vi "getElement.vi"(7 "Type and Defaults":variant, 8 "error in":errorcluster, 9 "pathList":string[](array[string]), 10 "basePath in":string, 11 "JSON String":string="{\n  \"VersionHistory\": {\n    \"InitialAuthor\": \"ABC\",\n    \"DateCreated\": \"03:45:56 AM 22/02/2017\",\n    \"DatesModified\": [\n      \"03:45:56 AM 22/02/2017\",\n      \"03:45:56 AM 22/02/2017\",\n      \"03:45:56 AM 22/02/2017\"\n    ],\n    \"ModifiedBy\": [\n      \"DEF\",\n      \"GHI\",\n      \"JKL\"\n    ],\n    \"DocumentVersion\": \"2.1.2\",\n    \"ZenParamsSpecVersion\": \"3.2.1\"\n  },\n  \"SystemParameters\": {\n    \"SystemName\": \"Tiger\",\n    \"SystemID\": 123,\n    \"CustomerName\": \"TT\",\n    \"Location\": \"Bangalore\",\n    \"InstallationDate\": \"10-02-2017\",\n    \"NextServiceDate\": \"16-07-2017\",\n    \"ServiceHistory\": [\n      \"16-07-2016\",\n      \"16-08-2016\"\n    ],\n    \"CompatibleZenGage\": \"1.1\",\n    \"TotalNumberOfCameras\": 3,\n    \"NumberOfRacks\": 1,\n    \"SoftwareFeature\": {\n      \"comment_SoftwareFeatures\": \"//Software feature contains controls to Enable/Disable POST, Cp Cpk Report, Analytics, Data Logging and control to set value for Maximum Digital Zoom//\",\n      \"POSTEnable\": true,\n      \"CpCpkReportEnable\": true,\n      \"AnalyticsEnable\": true,\n      \"DataLoggingEnable\": true,\n      \"MaxDigitalZoom\": 5\n    },\n    \"GuideHorizontalPositioningEnable\": true,\n    \"comment_Sensor\": \"//Sensor section contains Name, Unique Id, Controller IO number and Triggering Edge of each sensor//\",\n    \"Sensor\": [\n      {\n        \"Name\": \"pqr\",\n        \"Id\": 1,\n        \"ControllerIONumber\": 12,\n        \"Edge\": \"FALLING\"\n      },\n      {\n        \"Name\": \"stu\",\n        \"Id\": 2,\n        \"ControllerIONumber\": 12,\n        \"Edge\": \"FALLING\"\n      },\n      {\n        \"Name\": \"vwx\",\n        \"Id\": 3,\n        \"ControllerIONumber\": 12,\n        \"Edge\": \"FALLING\"\n      }\n    ],\n    \"comment_Light\": \"//Light section contains Name, Unique Id, Type (Can be Bright field, Dark field, Back light, Front light, Diffuse light, Co-Axial diffuse etc.), Controller IO number and Level (HIGH or LOW) of each Light//\",\n    \"Light\": [\n      {\n        \"Name\": \"Light1\",\n        \"Id\": 1,\n        \"Type\": \"Back\",\n        \"ControllerIONumber\": 23,\n        \"Level\": \"HIGH\"\n      },\n      {\n        \"Name\": \"Light2\",\n        \"Id\": 2,\n        \"Type\": \"Front\",\n        \"ControllerIONumber\": 23,\n        \"Level\": \"HIGH\"\n      },\n      {\n        \"Name\": \"Light3\",\n        \"Id\": 3,\n        \"Type\": \"Back\",\n        \"ControllerIONumber\": 23,\n        \"Level\": \"HIGH\"\n      }\n    ],\n    \"comment_Camera\": \"//Camera section contains Camera Id, Type (Top, Side or Front), Model, Area of Interest (AOI), Trigger Mode, Controller IO Number, Triggering Edge, Pulse Width, Exposure Time in micro seconds, Interface Type (Allowed values are USB3, GigE, USB2), Gain in dB, Calibration details (Date and file path) of each camera//\",\n    \"Camera\": [\n      {\n        \"Id\": 1,\n        \"Type\": \"Top\",\n        \"Model\": \"Basler Ace 5MP\",\n        \"AOI\": [\n          12,\n          34,\n          56,\n          78\n        ],\n        \"TriggerMode\": \"External\",\n        \"ControllerIONumber\": 34,\n        \"Edge\": \"FALLING\",\n        \"PulseWidth\": 233,\n        \"ExposureTimeUSec\": 12,\n        \"InterfaceType\": \"USB3\",\n        \"GainIndB\": 6,\n        \"CalibrationDate\": \"12-01-2017\",\n        \"CalibrationFilePath\": \"C:\\\\Users\\\\veenaj\\\\Desktop\"\n      },\n      {\n        \"Id\": 2,\n        \"Type\": \"Side\",\n        \"Model\": \"Basler Ace 5MP\",\n        \"AOI\": [\n          12,\n          34,\n          56,\n          78\n        ],\n        \"TriggerMode\": \"External\",\n        \"ControllerIONumber\": 34,\n        \"Edge\": \"FALLING\",\n        \"PulseWidth\": 233,\n        \"ExposureTimeUSec\": 12,\n        \"InterfaceType\": \"USB3\",\n        \"GainIndB\": 6,\n        \"CalibrationDate\": \"12/04/17\",\n        \"CalibrationFilePath\": \"C:\\\\Desktop\\\\Calibration\"\n      },\n      {\n        \"Id\": 3,\n        \"Type\": \"Front\",\n        \"Model\": \"Basler Ace 5MP\",\n        \"AOI\": [\n          12,\n          34,\n          56,\n          78\n        ],\n        \"TriggerMode\": \"External\",\n        \"ControllerIONumber\": 34,\n        \"Edge\": \"FALLING\",\n        \"PulseWidth\": 233,\n        \"ExposureTimeUSec\": 12,\n        \"InterfaceType\": \"USB3\",\n        \"GainIndB\": 6,\n        \"CalibrationDate\": \"12/04/17\",\n        \"CalibrationFilePath\": \"C:\\\\Desktop\\\\Calibration\"\n      }\n    ]\n  },\n  \"PartParameters\": {\n    \"comment_PartParameters\": \"//Parts Parameters section includes Number of Parts configured and Parts List. Part List contains Name, Parallel Trigger Threads, Number of measurements and Measurement details//\",\n    \"NumberOfPartsConfigured\": 2,\n    \"PartsList\": [\n      {\n        \"Name\": \"ECU1511\",\n        \"comment_ParallelTriggerThreads\": \"//ParallelTriggerThreads contain Thread Name, Thread Id and Imaging Views. Combination of Camera and Light(s) is defined in Imaging View along with Sensor to Light Delay (in micro seconds), Light to Camera Trigger Delay, Light Pulse Width and Reference Co-ordinate system. Each Imaging View is given a Name and unique ImageId. Camera and Light(s) are accessed by their unique Ids.//\",\n        \"ParallelTriggerThreads\": [\n          {\n            \"ThreadName\": \"TopRack\",\n            \"ThreadId\": 1,\n            \"ImagingViews\": [\n              {\n                \"ImageId\": 1,\n                \"ViewName\": \"TopProfileView\",\n                \"CameraId\": 3,\n                \"LightIds\": [\n                  1,\n                  4,\n                  5\n                ],\n                \"SensorToLightDelayinUSec\": 12,\n                \"LightToCameraTriggerDelay\": 24,\n                \"LightPulseWidth\": 123,\n                \"ReferenceCoordSystem\": {\n                  \"Method\": [\n                    \"A\",\n                    \"B\",\n                    \"C\",\n                    \"D\",\n                    \"R\",\n                    \"V\"\n                  ],\n                  \"comment_RefROI\": \"//Reference ROI is cluster of Left, Top, Right, Bottom and Rotation values//\",\n                  \"ROI1\": [\n                    1014,\n                    95,\n                    1290,\n                    520,\n                    0\n                  ],\n                  \"ROI2\": [\n                    740,\n                    70,\n                    1040,\n                    340,\n                    0\n                  ],\n                  \"ROI3\": [\n                    1060,\n                    88,\n                    723,\n                    85,\n                    0\n                  ],\n                  \"Name\": \"FirstReference\"\n                }\n              },\n              {\n                \"ImageId\": 2,\n                \"ViewName\": \"TopLightView\",\n                \"CameraId\": 2,\n                \"LightIds\": [\n                  2,\n                  3,\n                  5\n                ],\n                \"SensorToLightDelayinUSec\": 12,\n                \"LightToCameraTriggerDelay\": 24,\n                \"LightPulseWidth\": 123,\n                \"ReferenceCoordSystem\": {\n                  \"Method\": [\n                    \"A\",\n                    \"B\",\n                    \"C\",\n                    \"D\",\n                    \"R\",\n                    \"V\"\n                  ],\n                  \"comment_RefROI\": \"//Reference ROI is cluster of Left, Top, Right, Bottom and Rotation values//\",\n                  \"ROI1\": [\n                    1014,\n                    95,\n                    1290,\n                    520,\n                    0\n                  ],\n                  \"ROI2\": [\n                    740,\n                    70,\n                    1040,\n                    340,\n                    0\n                  ],\n                  \"ROI3\": [\n                    1060,\n                    88,\n                    723,\n                    85,\n                    0\n                  ],\n                  \"Name\": \"FirstReference\"\n                }\n              }\n            ]\n          },\n          {\n            \"ThreadName\": \"BottomRack\",\n            \"ThreadId\": 2,\n            \"ImagingViews\": [\n              {\n                \"ImageId\": 1,\n                \"ViewName\": \"TopProfileView\",\n                \"CameraId\": 3,\n                \"LightIds\": [\n                  1,\n                  4,\n                  5\n                ],\n                \"SensorToLightDelayinUSec\": 12,\n                \"LightToCameraTriggerDelay\": 24,\n                \"LightPulseWidth\": 123,\n                \"ReferenceCoordSystem\": {\n                  \"Method\": [\n                    \"A\",\n                    \"B\",\n                    \"C\",\n                    \"D\",\n                    \"R\",\n                    \"V\"\n                  ],\n                  \"comment_RefROI\": \"//Reference ROI is cluster of Left, Top, Right, Bottom and Rotation values//\",\n                  \"ROI1\": [\n                    1014,\n                    95,\n                    1290,\n                    520,\n                    0\n                  ],\n                  \"ROI2\": [\n                    740,\n                    70,\n                    1040,\n                    340,\n                    0\n                  ],\n                  \"ROI3\": [\n                    1060,\n                    88,\n                    723,\n                    85,\n                    0\n                  ],\n                  \"Name\": \"FirstReference\"\n                }\n              },\n              {\n                \"ImageId\": 2,\n                \"ViewName\": \"TopLightView\",\n                \"CameraId\": 2,\n                \"LightIds\": [\n                  2,\n                  3,\n                  5\n                ],\n                \"SensorToLightDelayinUSec\": 12,\n                \"LightToCameraTriggerDelay\": 24,\n                \"LightPulseWidth\": 123,\n                \"ReferenceCoordSystem\": {\n                  \"Method\": [\n                    \"A\",\n                    \"B\",\n                    \"C\",\n                    \"D\",\n                    \"R\",\n                    \"V\"\n                  ],\n                  \"comment_RefROI\": \"//Reference ROI is cluster of Left, Top, Right, Bottom and Rotation values//\",\n                  \"ROI1\": [\n                    1014,\n                    95,\n                    1290,\n                    520,\n                    0\n                  ],\n                  \"ROI2\": [\n                    740,\n                    70,\n                    1040,\n                    340,\n                    0\n                  ],\n                  \"ROI3\": [\n                    1060,\n                    88,\n                    723,\n                    85,\n                    0\n                  ],\n                  \"Name\": \"FirstReference\"\n                }\n              }\n            ]\n          },\n          {\n            \"ThreadName\": \"DentIdentification\",\n            \"ThreadId\": 3,\n            \"ImagingViews\": [\n              {\n                \"ImageId\": 1,\n                \"ViewName\": \"TopProfileView\",\n                \"CameraId\": 3,\n                \"LightIds\": [\n                  1,\n                  4,\n                  5\n                ],\n                \"SensorToLightDelayinUSec\": 12,\n                \"LightToCameraTriggerDelay\": 24,\n                \"LightPulseWidth\": 123,\n                \"ReferenceCoordSystem\": {\n                  \"Method\": [\n                    \"A\",\n                    \"B\",\n                    \"C\",\n                    \"D\",\n                    \"R\",\n                    \"V\"\n                  ],\n                  \"comment_RefROI\": \"//Reference ROI is cluster of Left, Top, Right, Bottom and Rotation values//\",\n                  \"ROI1\": [\n                    23,\n                    78,\n                    99,\n                    25,\n                    0\n                  ],\n                  \"ROI2\": [\n                    67,\n                    97,\n                    43,\n                    9,\n                    0\n                  ],\n                  \"ROI3\": [\n                    45,\n                    88,\n                    723,\n                    85,\n                    0\n                  ],\n                  \"Name\": \"FirstReference\"\n                }\n              }\n            ]\n          }\n        ],\n        \"Number of Measurements\": 3,\n        \"comment_Measurements\": \"//Measurements section contains Name, Type, Enable, Algorithm Sequence, Calibration Co-efficients, User Correction Linearity Coefficients, User Correction Bias Coefficients, LSL, USL, LCL, UCL, Control Limits Violation Threshold, Specification Limits Violation Threshold, Overlay Options, Datalog Enable, Display Icon path for each Measurement//\",\n        \"Measurements\": [\n          {\n            \"Name\": \"CollarWidth\",\n            \"comment_Type\": \"//Type can be Linear or Angle//\",\n            \"Type\": \"Linear\",\n            \"Enable\": true,\n            \"comment_AlgorithmSequence\": \"//Particular Measurement may require sequence of Algorithms. ThreadId and ThreadImageId are mentioned in each Algorithm which corresponds to particular combination of Camera and Light Ids. Result of each Algorithm is stored in a variable and final result is calculated using Math Expression defined.//\",\n            \"AlgorithmSequence\": [\n              {\n                \"AlgoName\": \"MaxClamp\",\n                \"ThreadId\": 1,\n                \"ThreadImageId\": 2,\n                \"Option1\": \"\",\n                \"Option2\": \"\",\n                \"Option3\": \"\",\n                \"LocalRef\": {\n                  \"LocalCoordinateSystemEnable\": true,\n                  \"Method\": [\n                    \"A\",\n                    \"B\",\n                    \"C\",\n                    \"D\",\n                    \"R\",\n                    \"V\"\n                  ],\n                  \"comment_LocalRefROI\": \"//Local Reference ROI is cluster of Left, Top, Right, Bottom and Rotation values//\",\n                  \"ROIs\": [\n                    [\n                      23,\n                      78,\n                      99,\n                      25,\n                      0\n                    ],\n                    [\n                      67,\n                      97,\n                      43,\n                      9,\n                      0\n                    ],\n                    [\n                      45,\n                      88,\n                      723,\n                      85,\n                      0\n                    ]\n                  ],\n                  \"Name\": \"CollarWidthLocalReference\"\n                },\n                \"LocalROIs\": [\n                  [\n                    23,\n                    78,\n                    99,\n                    25,\n                    0\n                  ],\n                  [\n                    67,\n                    97,\n                    43,\n                    9,\n                    0\n                  ],\n                  [\n                    45,\n                    88,\n                    723,\n                    85,\n                    0\n                  ]\n                ],\n                \"comment_Overlay\": \"//OverlayOptions contain Text, Co ordinates, Angle in Degrees, Text Size and Text Color for Overlay//\",\n                \"OverlayOptions\": {\n                  \"OverlayEnable\": true,\n                  \"OverlayText\": \"Collar Width\",\n                  \"OverlayCoords\": [\n                    5,\n                    8\n                  ],\n                  \"OverlayAngle\": 56,\n                  \"OverlayTextSize\": 6,\n                  \"OverlayTextColor\": \"Red\"\n                },\n                \"ResultVariable\": \"M1\"\n              },\n              {\n                \"AlgoName\": \"MoveXYTable\",\n                \"XYDelta\": [\n                  56,\n                  -33.8\n                ]\n              },\n              {\n                \"AlgoName\": \"MaxClamp\",\n                \"ThreadId\": 1,\n                \"ThreadImageId\": 2,\n                \"Option1\": \"\",\n                \"Option2\": \"\",\n                \"Option3\": \"\",\n                \"LocalRef\": {\n                  \"LocalCoordinateSystemEnable\": true,\n                  \"Method\": [\n                    \"A\",\n                    \"B\",\n                    \"C\",\n                    \"D\",\n                    \"R\",\n                    \"V\"\n                  ],\n                  \"ROIs\": [\n                    [\n                      23,\n                      78,\n                      99,\n                      25,\n                      0\n                    ],\n                    [\n                      67,\n                      97,\n                      43,\n                      9,\n                      0\n                    ],\n                    [\n                      45,\n                      88,\n                      723,\n                      85,\n                      0\n                    ]\n                  ],\n                  \"Name\": \"CollarWidthLocalReference\"\n                },\n                \"LocalROIs\": [\n                  [\n                    23,\n                    78,\n                    99,\n                    25,\n                    0\n                  ],\n                  [\n                    67,\n                    97,\n                    43,\n                    9,\n                    0\n                  ],\n                  [\n                    45,\n                    88,\n                    723,\n                    85,\n                    0\n                  ]\n                ],\n                \"comment_Overlay\": \"//OverlayOptions contain Text, Co ordinates, Angle in Degrees, Text Size and Text Color for Overlay//\",\n                \"OverlayOptions\": {\n                  \"OverlayEnable\": true,\n                  \"OverlayText\": \"Collar Width\",\n                  \"OverlayCoords\": [\n                    5,\n                    8\n                  ],\n                  \"OverlayAngle\": 56,\n                  \"OverlayTextSize\": 6,\n                  \"OverlayTextColor\": \"Red\"\n                },\n                \"ResultVariable\": \"M2\"\n              },\n              {\n                \"Algorithm\": \"Math\",\n                \"MathExpression\": \"M2-M1\",\n                \"ResultVariable\": \"M3\"\n              }\n            ],\n            \"CalibrationCoefficients\": [\n              13,\n              8.7,\n              67.9\n            ],\n            \"UserCorrectionLinearityCoeff\": 45,\n            \"UserCorrectionBiasCoeff\": 56,\n            \"comment_LSL\": \"//Lower Specification Limit//\",\n            \"LSL\": 13.5,\n            \"comment_USL\": \"//Upper Specification Limit//\",\n            \"USL\": 15,\n            \"comment_LCL\": \"//Lower Control Limit//\",\n            \"LCL\": 13.5,\n            \"comment_UCL\": \"//Upper Control Limit//\",\n            \"UCL\": 15,\n            \"comment_ControlLimitsViolationThreshold\": \"//If 3 measurement results out of 1000, are crossing LCL and UCL then fail is detected//\",\n            \"ControlLimitsViolationThreshold\": [\n              3,\n              1000\n            ],\n            \"comment_SpecificationLimitsViolationThreshold\": \"//If 5 measurement results out of 5000, are crossing LSL and USL then fail is detected//\",\n            \"SpecificationLimitViolationThreshold\": [\n              5,\n              5000\n            ],\n            \"comment_Overlay\": \"//OverlayOptions contain Text, Co ordinates, Angle in Degrees, Text Size and Text Color for Overlay//\",\n            \"OverlayOptions\": {\n              \"OverlayEnable\": true,\n              \"OverlayText\": \"Collar Width\",\n              \"OverlayCoords\": [\n                5,\n                8\n              ],\n              \"OverlayAngle\": 56,\n              \"OverlayTextSize\": 6,\n              \"OverlayTextColor\": \"Red\"\n            },\n            \"DatalogEnable\": true,\n            \"DisplayIcon\": \"C:\\\\Desktop\\\\displayimage.png\"\n          },\n          {\n            \"Name\": \"Length\",\n            \"comment_Type\": \"//Type can be Linear or Angle//\",\n            \"Type\": \"Linear\",\n            \"Enable\": true,\n            \"comment_AlgorithmSequence\": \"//Particular Measurement may require sequence of Algorithms. ThreadId and ThreadImageId are mentioned in each Algorithm which corresponds to particular combination of Camera and Light Ids. Result of each Algorithm is stored in a variable and final result is calculated using Math Expression defined.//\",\n            \"AlgorithmSequence\": [\n              {\n                \"AlgoName\": \"MaxClamp\",\n                \"ThreadId\": 1,\n                \"ThreadImageId\": 2,\n                \"Option1\": \"\",\n                \"Option2\": \"\",\n                \"Option3\": \"\",\n                \"LocalRef\": {\n                  \"LocalCoordinateSystemEnable\": true,\n                  \"Method\": [\n                    \"A\",\n                    \"B\",\n                    \"C\",\n                    \"D\",\n                    \"R\",\n                    \"V\"\n                  ],\n                  \"comment_LocalRefROI\": \"//Local Reference ROI is cluster of Left, Top, Right, Bottom and Rotation values//\",\n                  \"ROIs\": [\n                    [\n                      23,\n                      78,\n                      99,\n                      25,\n                      0\n                    ],\n                    [\n                      67,\n                      97,\n                      43,\n                      9,\n                      0\n                    ],\n                    [\n                      45,\n                      88,\n                      723,\n                      85,\n                      0\n                    ]\n                  ],\n                  \"Name\": \"CollarWidthLocalReference\"\n                },\n                \"LocalROIs\": [\n                  [\n                    23,\n                    78,\n                    99,\n                    25,\n                    0\n                  ],\n                  [\n                    67,\n                    97,\n                    43,\n                    9,\n                    0\n                  ],\n                  [\n                    45,\n                    88,\n                    723,\n                    85,\n                    0\n                  ]\n                ],\n                \"comment_Overlay\": \"//OverlayOptions contain Text, Co ordinates, Angle in Degrees, Text Size and Text Color for Overlay//\",\n                \"OverlayOptions\": {\n                  \"OverlayEnable\": true,\n                  \"OverlayText\": \"Collar Width\",\n                  \"OverlayCoords\": [\n                    5,\n                    8\n                  ],\n                  \"OverlayAngle\": 56,\n                  \"OverlayTextSize\": 6,\n                  \"OverlayTextColor\": \"Red\"\n                },\n                \"ResultVariable\": \"M1\"\n              },\n              {\n                \"AlgoName\": \"MoveXYTable\",\n                \"XYDelta\": [\n                  56,\n                  -33.8\n                ]\n              },\n              {\n                \"AlgoName\": \"MaxClamp\",\n                \"ThreadId\": 1,\n                \"ThreadImageId\": 2,\n                \"Option1\": \"\",\n                \"Option2\": \"\",\n                \"Option3\": \"\",\n                \"LocalRef\": {\n                  \"LocalCoordinateSystemEnable\": true,\n                  \"Method\": [\n                    \"A\",\n                    \"B\",\n                    \"C\",\n                    \"D\",\n                    \"R\",\n                    \"V\"\n                  ],\n                  \"ROIs\": [\n                    [\n                      23,\n                      78,\n                      99,\n                      25,\n                      0\n                    ],\n                    [\n                      67,\n                      97,\n                      43,\n                      9,\n                      0\n                    ],\n                    [\n                      45,\n                      88,\n                      723,\n                      85,\n                      0\n                    ]\n                  ],\n                  \"Name\": \"CollarWidthLocalReference\"\n                },\n                \"LocalROIs\": [\n                  [\n                    23,\n                    78,\n                    99,\n                    25,\n                    0\n                  ],\n                  [\n                    67,\n                    97,\n                    43,\n                    9,\n                    0\n                  ],\n                  [\n                    45,\n                    88,\n                    723,\n                    85,\n                    0\n                  ]\n                ],\n                \"comment_Overlay\": \"//OverlayOptions contain Text, Co ordinates, Angle in Degrees, Text Size and Text Color for Overlay//\",\n                \"OverlayOptions\": {\n                  \"OverlayEnable\": true,\n                  \"OverlayText\": \"Collar Width\",\n                  \"OverlayCoords\": [\n                    5,\n                    8\n                  ],\n                  \"OverlayAngle\": 56,\n                  \"OverlayTextSize\": 6,\n                  \"OverlayTextColor\": \"Red\"\n                },\n                \"ResultVariable\": \"M2\"\n              },\n              {\n                \"Algorithm\": \"Math\",\n                \"MathExpression\": \"M2-M1\",\n                \"ResultVariable\": \"M3\"\n              }\n            ],\n            \"CalibrationCoefficients\": [\n              13,\n              8.7,\n              67.9\n            ],\n            \"UserCorrectionLinearityCoeff\": 45,\n            \"UserCorrectionBiasCoeff\": 56,\n            \"comment_LSL\": \"//Lower Specification Limit//\",\n            \"LSL\": 13.5,\n            \"comment_USL\": \"//Upper Specification Limit//\",\n            \"USL\": 15,\n            \"comment_LCL\": \"//Lower Control Limit//\",\n            \"LCL\": 13.5,\n            \"comment_UCL\": \"//Upper Control Limit//\",\n            \"UCL\": 15,\n            \"comment_ControlLimitsViolationThreshold\": \"//If 3 measurement results out of 1000, are crossing LCL and UCL then fail is detected//\",\n            \"ControlLimitsViolationThreshold\": [\n              3,\n              1000\n            ],\n            \"comment_SpecificationLimitsViolationThreshold\": \"//If 5 measurement results out of 5000, are crossing LSL and USL then fail is detected//\",\n            \"SpecificationLimitViolationThreshold\": [\n              5,\n              5000\n            ],\n            \"comment_Overlay\": \"//OverlayOptions contain Text, Co ordinates, Angle in Degrees, Text Size and Text Color for Overlay//\",\n            \"OverlayOptions\": {\n              \"OverlayEnable\": true,\n              \"OverlayText\": \"Collar Width\",\n              \"OverlayCoords\": [\n                5,\n                8\n              ],\n              \"OverlayAngle\": 56,\n              \"OverlayTextSize\": 6,\n              \"OverlayTextColor\": \"Red\"\n            },\n            \"DatalogEnable\": true,\n            \"DisplayIcon\": \"C:\\\\Desktop\\\\displayimage.png\"\n          },\n          {\n            \"Name\": \"Length2\",\n            \"comment_Type\": \"//Type can be Linear or Angle//\",\n            \"Type\": \"Linear\",\n            \"Enable\": true,\n            \"comment_AlgorithmSequence\": \"//Particular Measurement may require sequence of Algorithms. ThreadId and ThreadImageId are mentioned in each Algorithm which corresponds to particular combination of Camera and Light Ids. Result of each Algorithm is stored in a variable and final result is calculated using Math Expression defined.//\",\n            \"AlgorithmSequence\": [\n              {\n                \"AlgoName\": \"MaxClamp\",\n                \"ThreadId\": 1,\n                \"ThreadImageId\": 2,\n                \"Option1\": \"\",\n                \"Option2\": \"\",\n                \"Option3\": \"\",\n                \"LocalRef\": {\n                  \"LocalCoordinateSystemEnable\": true,\n                  \"Method\": [\n                    \"A\",\n                    \"B\",\n                    \"C\",\n                    \"D\",\n                    \"R\",\n                    \"V\"\n                  ],\n                  \"comment_LocalRefROI\": \"//Local Reference ROI is cluster of Left, Top, Right, Bottom and Rotation values//\",\n                  \"ROIs\": [\n                    [\n                      23,\n                      78,\n                      99,\n                      25,\n                      0\n                    ],\n                    [\n                      67,\n                      97,\n                      43,\n                      9,\n                      0\n                    ],\n                    [\n                      45,\n                      88,\n                      723,\n                      85,\n                      0\n                    ]\n                  ],\n                  \"Name\": \"CollarWidthLocalReference\"\n                },\n                \"LocalROIs\": [\n                  [\n                    23,\n                    78,\n                    99,\n                    25,\n                    0\n                  ],\n                  [\n                    67,\n                    97,\n                    43,\n                    9,\n                    0\n                  ],\n                  [\n                    45,\n                    88,\n                    723,\n                    85,\n                    0\n                  ]\n                ],\n                \"comment_Overlay\": \"//OverlayOptions contain Text, Co ordinates, Angle in Degrees, Text Size and Text Color for Overlay//\",\n                \"OverlayOptions\": {\n                  \"OverlayEnable\": true,\n                  \"OverlayText\": \"Collar Width\",\n                  \"OverlayCoords\": [\n                    5,\n                    8\n                  ],\n                  \"OverlayAngle\": 56,\n                  \"OverlayTextSize\": 6,\n                  \"OverlayTextColor\": \"Red\"\n                },\n                \"ResultVariable\": \"M1\"\n              },\n              {\n                \"AlgoName\": \"MoveXYTable\",\n                \"XYDelta\": [\n                  56,\n                  -33.8\n                ]\n              },\n              {\n                \"AlgoName\": \"MaxClamp\",\n                \"ThreadId\": 1,\n                \"ThreadImageId\": 2,\n                \"Option1\": \"\",\n                \"Option2\": \"\",\n                \"Option3\": \"\",\n                \"LocalRef\": {\n                  \"LocalCoordinateSystemEnable\": true,\n                  \"Method\": [\n                    \"A\",\n                    \"B\",\n                    \"C\",\n                    \"D\",\n                    \"R\",\n                    \"V\"\n                  ],\n                  \"ROIs\": [\n                    [\n                      23,\n                      78,\n                      99,\n                      25,\n                      0\n                    ],\n                    [\n                      67,\n                      97,\n                      43,\n                      9,\n                      0\n                    ],\n                    [\n                      45,\n                      88,\n                      723,\n                      85,\n                      0\n                    ]\n                  ],\n                  \"Name\": \"CollarWidthLocalReference\"\n                },\n                \"LocalROIs\": [\n                  [\n                    23,\n                    78,\n                    99,\n                    25,\n                    0\n                  ],\n                  [\n                    67,\n                    97,\n                    43,\n                    9,\n                    0\n                  ],\n                  [\n                    45,\n                    88,\n                    723,\n                    85,\n                    0\n                  ]\n                ],\n                \"comment_Overlay\": \"//OverlayOptions contain Text, Co ordinates, Angle in Degrees, Text Size and Text Color for Overlay//\",\n                \"OverlayOptions\": {\n                  \"OverlayEnable\": true,\n                  \"OverlayText\": \"Collar Width\",\n                  \"OverlayCoords\": [\n                    5,\n                    8\n                  ],\n                  \"OverlayAngle\": 56,\n                  \"OverlayTextSize\": 6,\n                  \"OverlayTextColor\": \"Red\"\n                },\n                \"ResultVariable\": \"M2\"\n              },\n              {\n                \"Algorithm\": \"Math\",\n                \"MathExpression\": \"M2-M1\",\n                \"ResultVariable\": \"M3\"\n              }\n            ],\n            \"CalibrationCoefficients\": [\n              13,\n              8.7,\n              67.9\n            ],\n            \"UserCorrectionLinearityCoeff\": 45,\n            \"UserCorrectionBiasCoeff\": 56,\n            \"comment_LSL\": \"//Lower Specification Limit//\",\n            \"LSL\": 13.5,\n            \"comment_USL\": \"//Upper Specification Limit//\",\n            \"USL\": 15,\n            \"comment_LCL\": \"//Lower Control Limit//\",\n            \"LCL\": 13.5,\n            \"comment_UCL\": \"//Upper Control Limit//\",\n            \"UCL\": 15,\n            \"comment_ControlLimitsViolationThreshold\": \"//If 3 measurement results out of 1000, are crossing LCL and UCL then fail is detected//\",\n            \"ControlLimitsViolationThreshold\": [\n              3,\n              1000\n            ],\n            \"comment_SpecificationLimitsViolationThreshold\": \"//If 5 measurement results out of 5000, are crossing LSL and USL then fail is detected//\",\n            \"SpecificationLimitViolationThreshold\": [\n              5,\n              5000\n            ],\n            \"comment_Overlay\": \"//OverlayOptions contain Text, Co ordinates, Angle in Degrees, Text Size and Text Color for Overlay//\",\n            \"OverlayOptions\": {\n              \"OverlayEnable\": true,\n              \"OverlayText\": \"Collar Width\",\n              \"OverlayCoords\": [\n                5,\n                8\n              ],\n              \"OverlayAngle\": 56,\n              \"OverlayTextSize\": 6,\n              \"OverlayTextColor\": \"Red\"\n            },\n            \"DatalogEnable\": true,\n            \"DisplayIcon\": \"C:\\\\Desktop\\\\displayimage.png\"\n          }\n        ]\n      },\n      {\n        \"Name\": \"ECU1512\",\n        \"comment_ParallelTriggerThreads\": \"//ParallelTriggerThreads contain Thread Name, Thread Id and Imaging Views. Combination of Camera and Light(s) is defined in Imaging View along with Sensor to Light Delay (in micro seconds), Light to Camera Trigger Delay, Light Pulse Width and Reference Co-ordinate system. Each Imaging View is given a Name and unique ImageId. Camera and Light(s) are accessed by their unique Ids.//\",\n        \"ParallelTriggerThreads\": [\n          {\n            \"ThreadName\": \"TopRack\",\n            \"ThreadId\": 1,\n            \"ImagingViews\": [\n              {\n                \"ImageId\": 1,\n                \"ViewName\": \"TopProfileView\",\n                \"CameraId\": 3,\n                \"LightIds\": [\n                  1,\n                  4,\n                  5\n                ],\n                \"SensorToLightDelayinUSec\": 12,\n                \"LightToCameraTriggerDelay\": 24,\n                \"LightPulseWidth\": 123,\n                \"ReferenceCoordSystem\": {\n                  \"Method\": [\n                    \"A\",\n                    \"B\",\n                    \"C\",\n                    \"D\",\n                    \"R\",\n                    \"V\"\n                  ],\n                  \"comment_RefROI\": \"//Reference ROI is cluster of Left, Top, Right, Bottom and Rotation values//\",\n                  \"ROI1\": [\n                    1014,\n                    95,\n                    1290,\n                    520,\n                    0\n                  ],\n                  \"ROI2\": [\n                    740,\n                    70,\n                    1040,\n                    340,\n                    0\n                  ],\n                  \"ROI3\": [\n                    1060,\n                    88,\n                    723,\n                    85,\n                    0\n                  ],\n                  \"Name\": \"FirstReference\"\n                }\n              },\n              {\n                \"ImageId\": 2,\n                \"ViewName\": \"TopLightView\",\n                \"CameraId\": 2,\n                \"LightIds\": [\n                  2,\n                  3,\n                  5\n                ],\n                \"SensorToLightDelayinUSec\": 12,\n                \"LightToCameraTriggerDelay\": 24,\n                \"LightPulseWidth\": 123,\n                \"ReferenceCoordSystem\": {\n                  \"Method\": [\n                    \"A\",\n                    \"B\",\n                    \"C\",\n                    \"D\",\n                    \"R\",\n                    \"V\"\n                  ],\n                  \"comment_RefROI\": \"//Reference ROI is cluster of Left, Top, Right, Bottom and Rotation values//\",\n                  \"ROI1\": [\n                    1014,\n                    95,\n                    1290,\n                    520,\n                    0\n                  ],\n                  \"ROI2\": [\n                    740,\n                    70,\n                    1040,\n                    340,\n                    0\n                  ],\n                  \"ROI3\": [\n                    1060,\n                    88,\n                    723,\n                    85,\n                    0\n                  ],\n                  \"Name\": \"FirstReference\"\n                }\n              }\n            ]\n          },\n          {\n            \"ThreadName\": \"BottomRack\",\n            \"ThreadId\": 2,\n            \"ImagingViews\": [\n              {\n                \"ImageId\": 1,\n                \"ViewName\": \"TopProfileView\",\n                \"CameraId\": 3,\n                \"LightIds\": [\n                  1,\n                  4,\n                  5\n                ],\n                \"SensorToLightDelayinUSec\": 12,\n                \"LightToCameraTriggerDelay\": 24,\n                \"LightPulseWidth\": 123,\n                \"ReferenceCoordSystem\": {\n                  \"Method\": [\n                    \"A\",\n                    \"B\",\n                    \"C\",\n                    \"D\",\n                    \"R\",\n                    \"V\"\n                  ],\n                  \"comment_RefROI\": \"//Reference ROI is cluster of Left, Top, Right, Bottom and Rotation values//\",\n                  \"ROI1\": [\n                    1014,\n                    95,\n                    1290,\n                    520,\n                    0\n                  ],\n                  \"ROI2\": [\n                    740,\n                    70,\n                    1040,\n                    340,\n                    0\n                  ],\n                  \"ROI3\": [\n                    1060,\n                    88,\n                    723,\n                    85,\n                    0\n                  ],\n                  \"Name\": \"FirstReference\"\n                }\n              },\n              {\n                \"ImageId\": 2,\n                \"ViewName\": \"TopLightView\",\n                \"CameraId\": 2,\n                \"LightIds\": [\n                  2,\n                  3,\n                  5\n                ],\n                \"SensorToLightDelayinUSec\": 12,\n                \"LightToCameraTriggerDelay\": 24,\n                \"LightPulseWidth\": 123,\n                \"ReferenceCoordSystem\": {\n                  \"Method\": [\n                    \"A\",\n                    \"B\",\n                    \"C\",\n                    \"D\",\n                    \"R\",\n                    \"V\"\n                  ],\n                  \"comment_RefROI\": \"//Reference ROI is cluster of Left, Top, Right, Bottom and Rotation values//\",\n                  \"ROI1\": [\n                    1014,\n                    95,\n                    1290,\n                    520,\n                    0\n                  ],\n                  \"ROI2\": [\n                    740,\n                    70,\n                    1040,\n                    340,\n                    0\n                  ],\n                  \"ROI3\": [\n                    1060,\n                    88,\n                    723,\n                    85,\n                    0\n                  ],\n                  \"Name\": \"FirstReference\"\n                }\n              }\n            ]\n          },\n          {\n            \"ThreadName\": \"DentIdentification\",\n            \"ThreadId\": 3,\n            \"ImagingViews\": [\n              {\n                \"ImageId\": 1,\n                \"ViewName\": \"TopProfileView\",\n                \"CameraId\": 3,\n                \"LightIds\": [\n                  1,\n                  4,\n                  5\n                ],\n                \"SensorToLightDelayinUSec\": 12,\n                \"LightToCameraTriggerDelay\": 24,\n                \"LightPulseWidth\": 123,\n                \"ReferenceCoordSystem\": {\n                  \"Method\": [\n                    \"A\",\n                    \"B\",\n                    \"C\",\n                    \"D\",\n                    \"R\",\n                    \"V\"\n                  ],\n                  \"comment_RefROI\": \"//Reference ROI is cluster of Left, Top, Right, Bottom and Rotation values//\",\n                  \"ROI1\": [\n                    23,\n                    78,\n                    99,\n                    25,\n                    0\n                  ],\n                  \"ROI2\": [\n                    67,\n                    97,\n                    43,\n                    9,\n                    0\n                  ],\n                  \"ROI3\": [\n                    45,\n                    88,\n                    723,\n                    85,\n                    0\n                  ],\n                  \"Name\": \"FirstReference\"\n                }\n              }\n            ]\n          }\n        ],\n        \"comment_Measurements\": \"//Measurements section contains Name, Type, Enable, Algorithm Sequence, Calibration Co-efficients, User Correction Linearity Coefficients, User Correction Bias Coefficients, LSL, USL, LCL, UCL, Control Limits Violation Threshold, Specification Limits Violation Threshold, Overlay Options, Datalog Enable, Display Icon path for each Measurement//\",\n        \"Measurements\": [\n          {\n            \"Name\": \"CollarWidth\",\n            \"comment_Type\": \"//Type can be Linear or Angle//\",\n            \"Type\": \"Linear\",\n            \"Enable\": true,\n            \"comment_AlgorithmSequence\": \"//Particular Measurement may require sequence of Algorithms. ThreadId and ThreadImageId are mentioned in each Algorithm which corresponds to particular combination of Camera and Light Ids. Result of each Algorithm is stored in a variable and final result is calculated using Math Expression defined.//\",\n            \"AlgorithmSequence\": [\n              {\n                \"AlgoName\": \"MaxClamp\",\n                \"ThreadId\": 1,\n                \"ThreadImageId\": 2,\n                \"Option1\": \"\",\n                \"Option2\": \"\",\n                \"Option3\": \"\",\n                \"LocalRef\": {\n                  \"LocalCoordinateSystemEnable\": true,\n                  \"Method\": [\n                    \"A\",\n                    \"B\",\n                    \"C\",\n                    \"D\",\n                    \"R\",\n                    \"V\"\n                  ],\n                  \"comment_LocalRefROI\": \"//Local Reference ROI is cluster of Left, Top, Right, Bottom and Rotation values//\",\n                  \"ROIs\": [\n                    [\n                      23,\n                      78,\n                      99,\n                      25,\n                      0\n                    ],\n                    [\n                      67,\n                      97,\n                      43,\n                      9,\n                      0\n                    ],\n                    [\n                      45,\n                      88,\n                      723,\n                      85,\n                      0\n                    ]\n                  ],\n                  \"Name\": \"CollarWidthLocalReference\"\n                },\n                \"LocalROIs\": [\n                  [\n                    23,\n                    78,\n                    99,\n                    25,\n                    0\n                  ],\n                  [\n                    67,\n                    97,\n                    43,\n                    9,\n                    0\n                  ],\n                  [\n                    45,\n                    88,\n                    723,\n                    85,\n                    0\n                  ]\n                ],\n                \"comment_Overlay\": \"//OverlayOptions contain Text, Co ordinates, Angle in Degrees, Text Size and Text Color for Overlay//\",\n                \"OverlayOptions\": {\n                  \"OverlayEnable\": true,\n                  \"OverlayText\": \"Collar Width\",\n                  \"OverlayCoords\": [\n                    5,\n                    8\n                  ],\n                  \"OverlayAngle\": 56,\n                  \"OverlayTextSize\": 6,\n                  \"OverlayTextColor\": \"Red\"\n                },\n                \"ResultVariable\": \"M1\"\n              },\n              {\n                \"AlgoName\": \"MoveXYTable\",\n                \"XYDelta\": [\n                  56,\n                  -33.8\n                ]\n              },\n              {\n                \"AlgoName\": \"MaxClamp\",\n                \"ThreadId\": 1,\n                \"ThreadImageId\": 2,\n                \"Option1\": \"\",\n                \"Option2\": \"\",\n                \"Option3\": \"\",\n                \"LocalRef\": {\n                  \"LocalCoordinateSystemEnable\": true,\n                  \"Method\": [\n                    \"A\",\n                    \"B\",\n                    \"C\",\n                    \"D\",\n                    \"R\",\n                    \"V\"\n                  ],\n                  \"ROIs\": [\n                    [\n                      23,\n                      78,\n                      99,\n                      25,\n                      0\n                    ],\n                    [\n                      67,\n                      97,\n                      43,\n                      9,\n                      0\n                    ],\n                    [\n                      45,\n                      88,\n                      723,\n                      85,\n                      0\n                    ]\n                  ],\n                  \"Name\": \"CollarWidthLocalReference\"\n                },\n                \"LocalROIs\": [\n                  [\n                    23,\n                    78,\n                    99,\n                    25,\n                    0\n                  ],\n                  [\n                    67,\n                    97,\n                    43,\n                    9,\n                    0\n                  ],\n                  [\n                    45,\n                    88,\n                    723,\n                    85,\n                    0\n                  ]\n                ],\n                \"comment_Overlay\": \"//OverlayOptions contain Text, Co ordinates, Angle in Degrees, Text Size and Text Color for Overlay//\",\n                \"OverlayOptions\": {\n                  \"OverlayEnable\": true,\n                  \"OverlayText\": \"Collar Width\",\n                  \"OverlayCoords\": [\n                    5,\n                    8\n                  ],\n                  \"OverlayAngle\": 56,\n                  \"OverlayTextSize\": 6,\n                  \"OverlayTextColor\": \"Red\"\n                },\n                \"ResultVariable\": \"M2\"\n              },\n              {\n                \"Algorithm\": \"Math\",\n                \"MathExpression\": \"M2-M1\",\n                \"ResultVariable\": \"M3\"\n              }\n            ],\n            \"CalibrationCoefficients\": [\n              13,\n              8.7,\n              67.9\n            ],\n            \"UserCorrectionLinearityCoeff\": 45,\n            \"UserCorrectionBiasCoeff\": 56,\n            \"comment_LSL\": \"//Lower Specification Limit//\",\n            \"LSL\": 13.5,\n            \"comment_USL\": \"//Upper Specification Limit//\",\n            \"USL\": 15,\n            \"comment_LCL\": \"//Lower Control Limit//\",\n            \"LCL\": 13.5,\n            \"comment_UCL\": \"//Upper Control Limit//\",\n            \"UCL\": 15,\n            \"comment_ControlLimitsViolationThreshold\": \"//If 3 measurement results out of 1000, are crossing LCL and UCL then fail is detected//\",\n            \"ControlLimitsViolationThreshold\": [\n              3,\n              1000\n            ],\n            \"comment_SpecificationLimitsViolationThreshold\": \"//If 5 measurement results out of 5000, are crossing LSL and USL then fail is detected//\",\n            \"SpecificationLimitViolationThreshold\": [\n              5,\n              5000\n            ],\n            \"comment_Overlay\": \"//OverlayOptions contain Text, Co ordinates, Angle in Degrees, Text Size and Text Color for Overlay//\",\n            \"OverlayOptions\": {\n              \"OverlayEnable\": true,\n              \"OverlayText\": \"Collar Width\",\n              \"OverlayCoords\": [\n                5,\n                8\n              ],\n              \"OverlayAngle\": 56,\n              \"OverlayTextSize\": 6,\n              \"OverlayTextColor\": \"Red\"\n            },\n            \"DatalogEnable\": true,\n            \"DisplayIcon\": \"C:\\\\Desktop\\\\displayimage.png\"\n          },\n          {\n            \"Name\": \"Length\",\n            \"comment_Type\": \"//Type can be Linear or Angle//\",\n            \"Type\": \"Linear\",\n            \"Enable\": true,\n            \"comment_AlgorithmSequence\": \"//Particular Measurement may require sequence of Algorithms. ThreadId and ThreadImageId are mentioned in each Algorithm which corresponds to particular combination of Camera and Light Ids. Result of each Algorithm is stored in a variable and final result is calculated using Math Expression defined.//\",\n            \"AlgorithmSequence\": [\n              {\n                \"AlgoName\": \"MaxClamp\",\n                \"ThreadId\": 1,\n                \"ThreadImageId\": 2,\n                \"Option1\": \"\",\n                \"Option2\": \"\",\n                \"Option3\": \"\",\n                \"LocalRef\": {\n                  \"LocalCoordinateSystemEnable\": true,\n                  \"Method\": [\n                    \"A\",\n                    \"B\",\n                    \"C\",\n                    \"D\",\n                    \"R\",\n                    \"V\"\n                  ],\n                  \"comment_LocalRefROI\": \"//Local Reference ROI is cluster of Left, Top, Right, Bottom and Rotation values//\",\n                  \"ROIs\": [\n                    [\n                      23,\n                      78,\n                      99,\n                      25,\n                      0\n                    ],\n                    [\n                      67,\n                      97,\n                      43,\n                      9,\n                      0\n                    ],\n                    [\n                      45,\n                      88,\n                      723,\n                      85,\n                      0\n                    ]\n                  ],\n                  \"Name\": \"CollarWidthLocalReference\"\n                },\n                \"LocalROIs\": [\n                  [\n                    23,\n                    78,\n                    99,\n                    25,\n                    0\n                  ],\n                  [\n                    67,\n                    97,\n                    43,\n                    9,\n                    0\n                  ],\n                  [\n                    45,\n                    88,\n                    723,\n                    85,\n                    0\n                  ]\n                ],\n                \"comment_Overlay\": \"//OverlayOptions contain Text, Co ordinates, Angle in Degrees, Text Size and Text Color for Overlay//\",\n                \"OverlayOptions\": {\n                  \"OverlayEnable\": true,\n                  \"OverlayText\": \"Collar Width\",\n                  \"OverlayCoords\": [\n                    5,\n                    8\n                  ],\n                  \"OverlayAngle\": 56,\n                  \"OverlayTextSize\": 6,\n                  \"OverlayTextColor\": \"Red\"\n                },\n                \"ResultVariable\": \"M1\"\n              },\n              {\n                \"AlgoName\": \"MoveXYTable\",\n                \"XYDelta\": [\n                  56,\n                  -33.8\n                ]\n              },\n              {\n                \"AlgoName\": \"MaxClamp\",\n                \"ThreadId\": 1,\n                \"ThreadImageId\": 2,\n                \"Option1\": \"\",\n                \"Option2\": \"\",\n                \"Option3\": \"\",\n                \"LocalRef\": {\n                  \"LocalCoordinateSystemEnable\": true,\n                  \"Method\": [\n                    \"A\",\n                    \"B\",\n                    \"C\",\n                    \"D\",\n                    \"R\",\n                    \"V\"\n                  ],\n                  \"ROIs\": [\n                    [\n                      23,\n                      78,\n                      99,\n                      25,\n                      0\n                    ],\n                    [\n                      67,\n                      97,\n                      43,\n                      9,\n                      0\n                    ],\n                    [\n                      45,\n                      88,\n                      723,\n                      85,\n                      0\n                    ]\n                  ],\n                  \"Name\": \"CollarWidthLocalReference\"\n                },\n                \"LocalROIs\": [\n                  [\n                    23,\n                    78,\n                    99,\n                    25,\n                    0\n                  ],\n                  [\n                    67,\n                    97,\n                    43,\n                    9,\n                    0\n                  ],\n                  [\n                    45,\n                    88,\n                    723,\n                    85,\n                    0\n                  ]\n                ],\n                \"comment_Overlay\": \"//OverlayOptions contain Text, Co ordinates, Angle in Degrees, Text Size and Text Color for Overlay//\",\n                \"OverlayOptions\": {\n                  \"OverlayEnable\": true,\n                  \"OverlayText\": \"Collar Width\",\n                  \"OverlayCoords\": [\n                    5,\n                    8\n                  ],\n                  \"OverlayAngle\": 56,\n                  \"OverlayTextSize\": 6,\n                  \"OverlayTextColor\": \"Red\"\n                },\n                \"ResultVariable\": \"M2\"\n              },\n              {\n                \"Algorithm\": \"Math\",\n                \"MathExpression\": \"M2-M1\",\n                \"ResultVariable\": \"M3\"\n              }\n            ],\n            \"CalibrationCoefficients\": [\n              13,\n              8.7,\n              67.9\n            ],\n            \"UserCorrectionLinearityCoeff\": 45,\n            \"UserCorrectionBiasCoeff\": 56,\n            \"comment_LSL\": \"//Lower Specification Limit//\",\n            \"LSL\": 13.5,\n            \"comment_USL\": \"//Upper Specification Limit//\",\n            \"USL\": 15,\n            \"comment_LCL\": \"//Lower Control Limit//\",\n            \"LCL\": 13.5,\n            \"comment_UCL\": \"//Upper Control Limit//\",\n            \"UCL\": 15,\n            \"comment_ControlLimitsViolationThreshold\": \"//If 3 measurement results out of 1000, are crossing LCL and UCL then fail is detected//\",\n            \"ControlLimitsViolationThreshold\": [\n              3,\n              1000\n            ],\n            \"comment_SpecificationLimitsViolationThreshold\": \"//If 5 measurement results out of 5000, are crossing LSL and USL then fail is detected//\",\n            \"SpecificationLimitViolationThreshold\": [\n              5,\n              5000\n            ],\n            \"comment_Overlay\": \"//OverlayOptions contain Text, Co ordinates, Angle in Degrees, Text Size and Text Color for Overlay//\",\n            \"OverlayOptions\": {\n              \"OverlayEnable\": true,\n              \"OverlayText\": \"Collar Width\",\n              \"OverlayCoords\": [\n                5,\n                8\n              ],\n              \"OverlayAngle\": 56,\n              \"OverlayTextSize\": 6,\n              \"OverlayTextColor\": \"Red\"\n            },\n            \"DatalogEnable\": true,\n            \"DisplayIcon\": \"C:\\\\Desktop\\\\displayimage.png\"\n          },\n          {\n            \"Name\": \"Length2\",\n            \"comment_Type\": \"//Type can be Linear or Angle//\",\n            \"Type\": \"Linear\",\n            \"Enable\": true,\n            \"comment_AlgorithmSequence\": \"//Particular Measurement may require sequence of Algorithms. ThreadId and ThreadImageId are mentioned in each Algorithm which corresponds to particular combination of Camera and Light Ids. Result of each Algorithm is stored in a variable and final result is calculated using Math Expression defined.//\",\n            \"AlgorithmSequence\": [\n              {\n                \"AlgoName\": \"MaxClamp\",\n                \"ThreadId\": 1,\n                \"ThreadImageId\": 2,\n                \"Option1\": \"\",\n                \"Option2\": \"\",\n                \"Option3\": \"\",\n                \"LocalRef\": {\n                  \"LocalCoordinateSystemEnable\": true,\n                  \"Method\": [\n                    \"A\",\n                    \"B\",\n                    \"C\",\n                    \"D\",\n                    \"R\",\n                    \"V\"\n                  ],\n                  \"comment_LocalRefROI\": \"//Local Reference ROI is cluster of Left, Top, Right, Bottom and Rotation values//\",\n                  \"ROIs\": [\n                    [\n                      23,\n                      78,\n                      99,\n                      25,\n                      0\n                    ],\n                    [\n                      67,\n                      97,\n                      43,\n                      9,\n                      0\n                    ],\n                    [\n                      45,\n                      88,\n                      723,\n                      85,\n                      0\n                    ]\n                  ],\n                  \"Name\": \"CollarWidthLocalReference\"\n                },\n                \"LocalROIs\": [\n                  [\n                    23,\n                    78,\n                    99,\n                    25,\n                    0\n                  ],\n                  [\n                    67,\n                    97,\n                    43,\n                    9,\n                    0\n                  ],\n                  [\n                    45,\n                    88,\n                    723,\n                    85,\n                    0\n                  ]\n                ],\n                \"comment_Overlay\": \"//OverlayOptions contain Text, Co ordinates, Angle in Degrees, Text Size and Text Color for Overlay//\",\n                \"OverlayOptions\": {\n                  \"OverlayEnable\": true,\n                  \"OverlayText\": \"Collar Width\",\n                  \"OverlayCoords\": [\n                    5,\n                    8\n                  ],\n                  \"OverlayAngle\": 56,\n                  \"OverlayTextSize\": 6,\n                  \"OverlayTextColor\": \"Red\"\n                },\n                \"ResultVariable\": \"M1\"\n              },\n              {\n                \"AlgoName\": \"MoveXYTable\",\n                \"XYDelta\": [\n                  56,\n                  -33.8\n                ]\n              },\n              {\n                \"AlgoName\": \"MaxClamp\",\n                \"ThreadId\": 1,\n                \"ThreadImageId\": 2,\n                \"Option1\": \"\",\n                \"Option2\": \"\",\n                \"Option3\": \"\",\n                \"LocalRef\": {\n                  \"LocalCoordinateSystemEnable\": true,\n                  \"Method\": [\n                    \"A\",\n                    \"B\",\n                    \"C\",\n                    \"D\",\n                    \"R\",\n                    \"V\"\n                  ],\n                  \"ROIs\": [\n                    [\n                      23,\n                      78,\n                      99,\n                      25,\n                      0\n                    ],\n                    [\n                      67,\n                      97,\n                      43,\n                      9,\n                      0\n                    ],\n                    [\n                      45,\n                      88,\n                      723,\n                      85,\n                      0\n                    ]\n                  ],\n                  \"Name\": \"CollarWidthLocalReference\"\n                },\n                \"LocalROIs\": [\n                  [\n                    23,\n                    78,\n                    99,\n                    25,\n                    0\n                  ],\n                  [\n                    67,\n                    97,\n                    43,\n                    9,\n                    0\n                  ],\n                  [\n                    45,\n                    88,\n                    723,\n                    85,\n                    0\n                  ]\n                ],\n                \"comment_Overlay\": \"//OverlayOptions contain Text, Co ordinates, Angle in Degrees, Text Size and Text Color for Overlay//\",\n                \"OverlayOptions\": {\n                  \"OverlayEnable\": true,\n                  \"OverlayText\": \"Collar Width\",\n                  \"OverlayCoords\": [\n                    5,\n                    8\n                  ],\n                  \"OverlayAngle\": 56,\n                  \"OverlayTextSize\": 6,\n                  \"OverlayTextColor\": \"Red\"\n                },\n                \"ResultVariable\": \"M2\"\n              },\n              {\n                \"Algorithm\": \"Math\",\n                \"MathExpression\": \"M2-M1\",\n                \"ResultVariable\": \"M3\"\n              }\n            ],\n            \"CalibrationCoefficients\": [\n              13,\n              8.7,\n              67.9\n            ],\n            \"UserCorrectionLinearityCoeff\": 45,\n            \"UserCorrectionBiasCoeff\": 56,\n            \"comment_LSL\": \"//Lower Specification Limit//\",\n            \"LSL\": 13.5,\n            \"comment_USL\": \"//Upper Specification Limit//\",\n            \"USL\": 15,\n            \"comment_LCL\": \"//Lower Control Limit//\",\n            \"LCL\": 13.5,\n            \"comment_UCL\": \"//Upper Control Limit//\",\n            \"UCL\": 15,\n            \"comment_ControlLimitsViolationThreshold\": \"//If 3 measurement results out of 1000, are crossing LCL and UCL then fail is detected//\",\n            \"ControlLimitsViolationThreshold\": [\n              3,\n              1000\n            ],\n            \"comment_SpecificationLimitsViolationThreshold\": \"//If 5 measurement results out of 5000, are crossing LSL and USL then fail is detected//\",\n            \"SpecificationLimitViolationThreshold\": [\n              5,\n              5000\n            ],\n            \"comment_Overlay\": \"//OverlayOptions contain Text, Co ordinates, Angle in Degrees, Text Size and Text Color for Overlay//\",\n            \"OverlayOptions\": {\n              \"OverlayEnable\": true,\n              \"OverlayText\": \"Collar Width\",\n              \"OverlayCoords\": [\n                5,\n                8\n              ],\n              \"OverlayAngle\": 56,\n              \"OverlayTextSize\": 6,\n              \"OverlayTextColor\": \"Red\"\n            },\n            \"DatalogEnable\": true,\n            \"DisplayIcon\": \"C:\\\\Desktop\\\\displayimage.png\"\n          }\n        ]\n      },\n      {\n        \"Name\": \"ECU1513\",\n        \"comment_ParallelTriggerThreads\": \"//ParallelTriggerThreads contain Thread Name, Thread Id and Imaging Views. Combination of Camera and Light(s) is defined in Imaging View along with Sensor to Light Delay (in micro seconds), Light to Camera Trigger Delay, Light Pulse Width and Reference Co-ordinate system. Each Imaging View is given a Name and unique ImageId. Camera and Light(s) are accessed by their unique Ids.//\",\n        \"ParallelTriggerThreads\": [\n          {\n            \"ThreadName\": \"TopRack\",\n            \"ThreadId\": 1,\n            \"ImagingViews\": [\n              {\n                \"ImageId\": 1,\n                \"ViewName\": \"TopProfileView\",\n                \"CameraId\": 3,\n                \"LightIds\": [\n                  1,\n                  4,\n                  5\n                ],\n                \"SensorToLightDelayinUSec\": 12,\n                \"LightToCameraTriggerDelay\": 24,\n                \"LightPulseWidth\": 123,\n                \"ReferenceCoordSystem\": {\n                  \"Method\": [\n                    \"A\",\n                    \"B\",\n                    \"C\",\n                    \"D\",\n                    \"R\",\n                    \"V\"\n                  ],\n                  \"comment_RefROI\": \"//Reference ROI is cluster of Left, Top, Right, Bottom and Rotation values//\",\n                  \"ROI1\": [\n                    1014,\n                    95,\n                    1290,\n                    520,\n                    0\n                  ],\n                  \"ROI2\": [\n                    740,\n                    70,\n                    1040,\n                    340,\n                    0\n                  ],\n                  \"ROI3\": [\n                    1060,\n                    88,\n                    723,\n                    85,\n                    0\n                  ],\n                  \"Name\": \"FirstReference\"\n                }\n              },\n              {\n                \"ImageId\": 2,\n                \"ViewName\": \"TopLightView\",\n                \"CameraId\": 2,\n                \"LightIds\": [\n                  2,\n                  3,\n                  5\n                ],\n                \"SensorToLightDelayinUSec\": 12,\n                \"LightToCameraTriggerDelay\": 24,\n                \"LightPulseWidth\": 123,\n                \"ReferenceCoordSystem\": {\n                  \"Method\": [\n                    \"A\",\n                    \"B\",\n                    \"C\",\n                    \"D\",\n                    \"R\",\n                    \"V\"\n                  ],\n                  \"comment_RefROI\": \"//Reference ROI is cluster of Left, Top, Right, Bottom and Rotation values//\",\n                  \"ROI1\": [\n                    1014,\n                    95,\n                    1290,\n                    520,\n                    0\n                  ],\n                  \"ROI2\": [\n                    740,\n                    70,\n                    1040,\n                    340,\n                    0\n                  ],\n                  \"ROI3\": [\n                    1060,\n                    88,\n                    723,\n                    85,\n                    0\n                  ],\n                  \"Name\": \"FirstReference\"\n                }\n              }\n            ]\n          },\n          {\n            \"ThreadName\": \"BottomRack\",\n            \"ThreadId\": 2,\n            \"ImagingViews\": [\n              {\n                \"ImageId\": 1,\n                \"ViewName\": \"TopProfileView\",\n                \"CameraId\": 3,\n                \"LightIds\": [\n                  1,\n                  4,\n                  5\n                ],\n                \"SensorToLightDelayinUSec\": 12,\n                \"LightToCameraTriggerDelay\": 24,\n                \"LightPulseWidth\": 123,\n                \"ReferenceCoordSystem\": {\n                  \"Method\": [\n                    \"A\",\n                    \"B\",\n                    \"C\",\n                    \"D\",\n                    \"R\",\n                    \"V\"\n                  ],\n                  \"comment_RefROI\": \"//Reference ROI is cluster of Left, Top, Right, Bottom and Rotation values//\",\n                  \"ROI1\": [\n                    1014,\n                    95,\n                    1290,\n                    520,\n                    0\n                  ],\n                  \"ROI2\": [\n                    740,\n                    70,\n                    1040,\n                    340,\n                    0\n                  ],\n                  \"ROI3\": [\n                    1060,\n                    88,\n                    723,\n                    85,\n                    0\n                  ],\n                  \"Name\": \"FirstReference\"\n                }\n              },\n              {\n                \"ImageId\": 2,\n                \"ViewName\": \"TopLightView\",\n                \"CameraId\": 2,\n                \"LightIds\": [\n                  2,\n                  3,\n                  5\n                ],\n                \"SensorToLightDelayinUSec\": 12,\n                \"LightToCameraTriggerDelay\": 24,\n                \"LightPulseWidth\": 123,\n                \"ReferenceCoordSystem\": {\n                  \"Method\": [\n                    \"A\",\n                    \"B\",\n                    \"C\",\n                    \"D\",\n                    \"R\",\n                    \"V\"\n                  ],\n                  \"comment_RefROI\": \"//Reference ROI is cluster of Left, Top, Right, Bottom and Rotation values//\",\n                  \"ROI1\": [\n                    1014,\n                    95,\n                    1290,\n                    520,\n                    0\n                  ],\n                  \"ROI2\": [\n                    740,\n                    70,\n                    1040,\n                    340,\n                    0\n                  ],\n                  \"ROI3\": [\n                    1060,\n                    88,\n                    723,\n                    85,\n                    0\n                  ],\n                  \"Name\": \"FirstReference\"\n                }\n              }\n            ]\n          },\n          {\n            \"ThreadName\": \"DentIdentification\",\n            \"ThreadId\": 3,\n            \"ImagingViews\": [\n              {\n                \"ImageId\": 1,\n                \"ViewName\": \"TopProfileView\",\n                \"CameraId\": 3,\n                \"LightIds\": [\n                  1,\n                  4,\n                  5\n                ],\n                \"SensorToLightDelayinUSec\": 12,\n                \"LightToCameraTriggerDelay\": 24,\n                \"LightPulseWidth\": 123,\n                \"ReferenceCoordSystem\": {\n                  \"Method\": [\n                    \"A\",\n                    \"B\",\n                    \"C\",\n                    \"D\",\n                    \"R\",\n                    \"V\"\n                  ],\n                  \"comment_RefROI\": \"//Reference ROI is cluster of Left, Top, Right, Bottom and Rotation values//\",\n                  \"ROI1\": [\n                    23,\n                    78,\n                    99,\n                    25,\n                    0\n                  ],\n                  \"ROI2\": [\n                    67,\n                    97,\n                    43,\n                    9,\n                    0\n                  ],\n                  \"ROI3\": [\n                    45,\n                    88,\n                    723,\n                    85,\n                    0\n                  ],\n                  \"Name\": \"FirstReference\"\n                }\n              }\n            ]\n          }\n        ],\n        \"Number of Measurements\": 3,\n        \"comment_Measurements\": \"//Measurements section contains Name, Type, Enable, Algorithm Sequence, Calibration Co-efficients, User Correction Linearity Coefficients, User Correction Bias Coefficients, LSL, USL, LCL, UCL, Control Limits Violation Threshold, Specification Limits Violation Threshold, Overlay Options, Datalog Enable, Display Icon path for each Measurement//\",\n        \"Measurements\": [\n          {\n            \"Name\": \"CollarWidth\",\n            \"comment_Type\": \"//Type can be Linear or Angle//\",\n            \"Type\": \"Linear\",\n            \"Enable\": true,\n            \"comment_AlgorithmSequence\": \"//Particular Measurement may require sequence of Algorithms. ThreadId and ThreadImageId are mentioned in each Algorithm which corresponds to particular combination of Camera and Light Ids. Result of each Algorithm is stored in a variable and final result is calculated using Math Expression defined.//\",\n            \"AlgorithmSequence\": [\n              {\n                \"AlgoName\": \"MaxClamp\",\n                \"ThreadId\": 1,\n                \"ThreadImageId\": 2,\n                \"Option1\": \"\",\n                \"Option2\": \"\",\n                \"Option3\": \"\",\n                \"LocalRef\": {\n                  \"LocalCoordinateSystemEnable\": true,\n                  \"Method\": [\n                    \"A\",\n                    \"B\",\n                    \"C\",\n                    \"D\",\n                    \"R\",\n                    \"V\"\n                  ],\n                  \"comment_LocalRefROI\": \"//Local Reference ROI is cluster of Left, Top, Right, Bottom and Rotation values//\",\n                  \"ROIs\": [\n                    [\n                      23,\n                      78,\n                      99,\n                      25,\n                      0\n                    ],\n                    [\n                      67,\n                      97,\n                      43,\n                      9,\n                      0\n                    ],\n                    [\n                      45,\n                      88,\n                      723,\n                      85,\n                      0\n                    ]\n                  ],\n                  \"Name\": \"CollarWidthLocalReference\"\n                },\n                \"LocalROIs\": [\n                  [\n                    23,\n                    78,\n                    99,\n                    25,\n                    0\n                  ],\n                  [\n                    67,\n                    97,\n                    43,\n                    9,\n                    0\n                  ],\n                  [\n                    45,\n                    88,\n                    723,\n                    85,\n                    0\n                  ]\n                ],\n                \"comment_Overlay\": \"//OverlayOptions contain Text, Co ordinates, Angle in Degrees, Text Size and Text Color for Overlay//\",\n                \"OverlayOptions\": {\n                  \"OverlayEnable\": true,\n                  \"OverlayText\": \"Collar Width\",\n                  \"OverlayCoords\": [\n                    5,\n                    8\n                  ],\n                  \"OverlayAngle\": 56,\n                  \"OverlayTextSize\": 6,\n                  \"OverlayTextColor\": \"Red\"\n                },\n                \"ResultVariable\": \"M1\"\n              },\n              {\n                \"AlgoName\": \"MoveXYTable\",\n                \"XYDelta\": [\n                  56,\n                  -33.8\n                ]\n              },\n              {\n                \"AlgoName\": \"MaxClamp\",\n                \"ThreadId\": 1,\n                \"ThreadImageId\": 2,\n                \"Option1\": \"\",\n                \"Option2\": \"\",\n                \"Option3\": \"\",\n                \"LocalRef\": {\n                  \"LocalCoordinateSystemEnable\": true,\n                  \"Method\": [\n                    \"A\",\n                    \"B\",\n                    \"C\",\n                    \"D\",\n                    \"R\",\n                    \"V\"\n                  ],\n                  \"ROIs\": [\n                    [\n                      23,\n                      78,\n                      99,\n                      25,\n                      0\n                    ],\n                    [\n                      67,\n                      97,\n                      43,\n                      9,\n                      0\n                    ],\n                    [\n                      45,\n                      88,\n                      723,\n                      85,\n                      0\n                    ]\n                  ],\n                  \"Name\": \"CollarWidthLocalReference\"\n                },\n                \"LocalROIs\": [\n                  [\n                    23,\n                    78,\n                    99,\n                    25,\n                    0\n                  ],\n                  [\n                    67,\n                    97,\n                    43,\n                    9,\n                    0\n                  ],\n                  [\n                    45,\n                    88,\n                    723,\n                    85,\n                    0\n                  ]\n                ],\n                \"comment_Overlay\": \"//OverlayOptions contain Text, Co ordinates, Angle in Degrees, Text Size and Text Color for Overlay//\",\n                \"OverlayOptions\": {\n                  \"OverlayEnable\": true,\n                  \"OverlayText\": \"Collar Width\",\n                  \"OverlayCoords\": [\n                    5,\n                    8\n                  ],\n                  \"OverlayAngle\": 56,\n                  \"OverlayTextSize\": 6,\n                  \"OverlayTextColor\": \"Red\"\n                },\n                \"ResultVariable\": \"M2\"\n              },\n              {\n                \"Algorithm\": \"Math\",\n                \"MathExpression\": \"M2-M1\",\n                \"ResultVariable\": \"M3\"\n              }\n            ],\n            \"CalibrationCoefficients\": [\n              13,\n              8.7,\n              67.9\n            ],\n            \"UserCorrectionLinearityCoeff\": 45,\n            \"UserCorrectionBiasCoeff\": 56,\n            \"comment_LSL\": \"//Lower Specification Limit//\",\n            \"LSL\": 13.5,\n            \"comment_USL\": \"//Upper Specification Limit//\",\n            \"USL\": 15,\n            \"comment_LCL\": \"//Lower Control Limit//\",\n            \"LCL\": 13.5,\n            \"comment_UCL\": \"//Upper Control Limit//\",\n            \"UCL\": 15,\n            \"comment_ControlLimitsViolationThreshold\": \"//If 3 measurement results out of 1000, are crossing LCL and UCL then fail is detected//\",\n            \"ControlLimitsViolationThreshold\": [\n              3,\n              1000\n            ],\n            \"comment_SpecificationLimitsViolationThreshold\": \"//If 5 measurement results out of 5000, are crossing LSL and USL then fail is detected//\",\n            \"SpecificationLimitViolationThreshold\": [\n              5,\n              5000\n            ],\n            \"comment_Overlay\": \"//OverlayOptions contain Text, Co ordinates, Angle in Degrees, Text Size and Text Color for Overlay//\",\n            \"OverlayOptions\": {\n              \"OverlayEnable\": true,\n              \"OverlayText\": \"Collar Width\",\n              \"OverlayCoords\": [\n                5,\n                8\n              ],\n              \"OverlayAngle\": 56,\n              \"OverlayTextSize\": 6,\n              \"OverlayTextColor\": \"Red\"\n            },\n            \"DatalogEnable\": true,\n            \"DisplayIcon\": \"C:\\\\Desktop\\\\displayimage.png\"\n          },\n          {\n            \"Name\": \"Length\",\n            \"comment_Type\": \"//Type can be Linear or Angle//\",\n            \"Type\": \"Linear\",\n            \"Enable\": true,\n            \"comment_AlgorithmSequence\": \"//Particular Measurement may require sequence of Algorithms. ThreadId and ThreadImageId are mentioned in each Algorithm which corresponds to particular combination of Camera and Light Ids. Result of each Algorithm is stored in a variable and final result is calculated using Math Expression defined.//\",\n            \"AlgorithmSequence\": [\n              {\n                \"AlgoName\": \"MaxClamp\",\n                \"ThreadId\": 1,\n                \"ThreadImageId\": 2,\n                \"Option1\": \"\",\n                \"Option2\": \"\",\n                \"Option3\": \"\",\n                \"LocalRef\": {\n                  \"LocalCoordinateSystemEnable\": true,\n                  \"Method\": [\n                    \"A\",\n                    \"B\",\n                    \"C\",\n                    \"D\",\n                    \"R\",\n                    \"V\"\n                  ],\n                  \"comment_LocalRefROI\": \"//Local Reference ROI is cluster of Left, Top, Right, Bottom and Rotation values//\",\n                  \"ROIs\": [\n                    [\n                      23,\n                      78,\n                      99,\n                      25,\n                      0\n                    ],\n                    [\n                      67,\n                      97,\n                      43,\n                      9,\n                      0\n                    ],\n                    [\n                      45,\n                      88,\n                      723,\n                      85,\n                      0\n                    ]\n                  ],\n                  \"Name\": \"CollarWidthLocalReference\"\n                },\n                \"LocalROIs\": [\n                  [\n                    23,\n                    78,\n                    99,\n                    25,\n                    0\n                  ],\n                  [\n                    67,\n                    97,\n                    43,\n                    9,\n                    0\n                  ],\n                  [\n                    45,\n                    88,\n                    723,\n                    85,\n                    0\n                  ]\n                ],\n                \"comment_Overlay\": \"//OverlayOptions contain Text, Co ordinates, Angle in Degrees, Text Size and Text Color for Overlay//\",\n                \"OverlayOptions\": {\n                  \"OverlayEnable\": true,\n                  \"OverlayText\": \"Collar Width\",\n                  \"OverlayCoords\": [\n                    5,\n                    8\n                  ],\n                  \"OverlayAngle\": 56,\n                  \"OverlayTextSize\": 6,\n                  \"OverlayTextColor\": \"Red\"\n                },\n                \"ResultVariable\": \"M1\"\n              },\n              {\n                \"AlgoName\": \"MoveXYTable\",\n                \"XYDelta\": [\n                  56,\n                  -33.8\n                ]\n              },\n              {\n                \"AlgoName\": \"MaxClamp\",\n                \"ThreadId\": 1,\n                \"ThreadImageId\": 2,\n                \"Option1\": \"\",\n                \"Option2\": \"\",\n                \"Option3\": \"\",\n                \"LocalRef\": {\n                  \"LocalCoordinateSystemEnable\": true,\n                  \"Method\": [\n                    \"A\",\n                    \"B\",\n                    \"C\",\n                    \"D\",\n                    \"R\",\n                    \"V\"\n                  ],\n                  \"ROIs\": [\n                    [\n                      23,\n                      78,\n                      99,\n                      25,\n                      0\n                    ],\n                    [\n                      67,\n                      97,\n                      43,\n                      9,\n                      0\n                    ],\n                    [\n                      45,\n                      88,\n                      723,\n                      85,\n                      0\n                    ]\n                  ],\n                  \"Name\": \"CollarWidthLocalReference\"\n                },\n                \"LocalROIs\": [\n                  [\n                    23,\n                    78,\n                    99,\n                    25,\n                    0\n                  ],\n                  [\n                    67,\n                    97,\n                    43,\n                    9,\n                    0\n                  ],\n                  [\n                    45,\n                    88,\n                    723,\n                    85,\n                    0\n                  ]\n                ],\n                \"comment_Overlay\": \"//OverlayOptions contain Text, Co ordinates, Angle in Degrees, Text Size and Text Color for Overlay//\",\n                \"OverlayOptions\": {\n                  \"OverlayEnable\": true,\n                  \"OverlayText\": \"Collar Width\",\n                  \"OverlayCoords\": [\n                    5,\n                    8\n                  ],\n                  \"OverlayAngle\": 56,\n                  \"OverlayTextSize\": 6,\n                  \"OverlayTextColor\": \"Red\"\n                },\n                \"ResultVariable\": \"M2\"\n              },\n              {\n                \"Algorithm\": \"Math\",\n                \"MathExpression\": \"M2-M1\",\n                \"ResultVariable\": \"M3\"\n              }\n            ],\n            \"CalibrationCoefficients\": [\n              13,\n              8.7,\n              67.9\n            ],\n            \"UserCorrectionLinearityCoeff\": 45,\n            \"UserCorrectionBiasCoeff\": 56,\n            \"comment_LSL\": \"//Lower Specification Limit//\",\n            \"LSL\": 13.5,\n            \"comment_USL\": \"//Upper Specification Limit//\",\n            \"USL\": 15,\n            \"comment_LCL\": \"//Lower Control Limit//\",\n            \"LCL\": 13.5,\n            \"comment_UCL\": \"//Upper Control Limit//\",\n            \"UCL\": 15,\n            \"comment_ControlLimitsViolationThreshold\": \"//If 3 measurement results out of 1000, are crossing LCL and UCL then fail is detected//\",\n            \"ControlLimitsViolationThreshold\": [\n              3,\n              1000\n            ],\n            \"comment_SpecificationLimitsViolationThreshold\": \"//If 5 measurement results out of 5000, are crossing LSL and USL then fail is detected//\",\n            \"SpecificationLimitViolationThreshold\": [\n              5,\n              5000\n            ],\n            \"comment_Overlay\": \"//OverlayOptions contain Text, Co ordinates, Angle in Degrees, Text Size and Text Color for Overlay//\",\n            \"OverlayOptions\": {\n              \"OverlayEnable\": true,\n              \"OverlayText\": \"Collar Width\",\n              \"OverlayCoords\": [\n                5,\n                8\n              ],\n              \"OverlayAngle\": 56,\n              \"OverlayTextSize\": 6,\n              \"OverlayTextColor\": \"Red\"\n            },\n            \"DatalogEnable\": true,\n            \"DisplayIcon\": \"C:\\\\Desktop\\\\displayimage.png\"\n          },\n          {\n            \"Name\": \"Length2\",\n            \"comment_Type\": \"//Type can be Linear or Angle//\",\n            \"Type\": \"Linear\",\n            \"Enable\": true,\n            \"comment_AlgorithmSequence\": \"//Particular Measurement may require sequence of Algorithms. ThreadId and ThreadImageId are mentioned in each Algorithm which corresponds to particular combination of Camera and Light Ids. Result of each Algorithm is stored in a variable and final result is calculated using Math Expression defined.//\",\n            \"AlgorithmSequence\": [\n              {\n                \"AlgoName\": \"MaxClamp\",\n                \"ThreadId\": 1,\n                \"ThreadImageId\": 2,\n                \"Option1\": \"\",\n                \"Option2\": \"\",\n                \"Option3\": \"\",\n                \"LocalRef\": {\n                  \"LocalCoordinateSystemEnable\": true,\n                  \"Method\": [\n                    \"A\",\n                    \"B\",\n                    \"C\",\n                    \"D\",\n                    \"R\",\n                    \"V\"\n                  ],\n                  \"comment_LocalRefROI\": \"//Local Reference ROI is cluster of Left, Top, Right, Bottom and Rotation values//\",\n                  \"ROIs\": [\n                    [\n                      23,\n                      78,\n                      99,\n                      25,\n                      0\n                    ],\n                    [\n                      67,\n                      97,\n                      43,\n                      9,\n                      0\n                    ],\n                    [\n                      45,\n                      88,\n                      723,\n                      85,\n                      0\n                    ]\n                  ],\n                  \"Name\": \"CollarWidthLocalReference\"\n                },\n                \"LocalROIs\": [\n                  [\n                    23,\n                    78,\n                    99,\n                    25,\n                    0\n                  ],\n                  [\n                    67,\n                    97,\n                    43,\n                    9,\n                    0\n                  ],\n                  [\n                    45,\n                    88,\n                    723,\n                    85,\n                    0\n                  ]\n                ],\n                \"comment_Overlay\": \"//OverlayOptions contain Text, Co ordinates, Angle in Degrees, Text Size and Text Color for Overlay//\",\n                \"OverlayOptions\": {\n                  \"OverlayEnable\": true,\n                  \"OverlayText\": \"Collar Width\",\n                  \"OverlayCoords\": [\n                    5,\n                    8\n                  ],\n                  \"OverlayAngle\": 56,\n                  \"OverlayTextSize\": 6,\n                  \"OverlayTextColor\": \"Red\"\n                },\n                \"ResultVariable\": \"M1\"\n              },\n              {\n                \"AlgoName\": \"MoveXYTable\",\n                \"XYDelta\": [\n                  56,\n                  -33.8\n                ]\n              },\n              {\n                \"AlgoName\": \"MaxClamp\",\n                \"ThreadId\": 1,\n                \"ThreadImageId\": 2,\n                \"Option1\": \"\",\n                \"Option2\": \"\",\n                \"Option3\": \"\",\n                \"LocalRef\": {\n                  \"LocalCoordinateSystemEnable\": true,\n                  \"Method\": [\n                    \"A\",\n                    \"B\",\n                    \"C\",\n                    \"D\",\n                    \"R\",\n                    \"V\"\n                  ],\n                  \"ROIs\": [\n                    [\n                      23,\n                      78,\n                      99,\n                      25,\n                      0\n                    ],\n                    [\n                      67,\n                      97,\n                      43,\n                      9,\n                      0\n                    ],\n                    [\n                      45,\n                      88,\n                      723,\n                      85,\n                      0\n                    ]\n                  ],\n                  \"Name\": \"CollarWidthLocalReference\"\n                },\n                \"LocalROIs\": [\n                  [\n                    23,\n                    78,\n                    99,\n                    25,\n                    0\n                  ],\n                  [\n                    67,\n                    97,\n                    43,\n                    9,\n                    0\n                  ],\n                  [\n                    45,\n                    88,\n                    723,\n                    85,\n                    0\n                  ]\n                ],\n                \"comment_Overlay\": \"//OverlayOptions contain Text, Co ordinates, Angle in Degrees, Text Size and Text Color for Overlay//\",\n                \"OverlayOptions\": {\n                  \"OverlayEnable\": true,\n                  \"OverlayText\": \"Collar Width\",\n                  \"OverlayCoords\": [\n                    5,\n                    8\n                  ],\n                  \"OverlayAngle\": 56,\n                  \"OverlayTextSize\": 6,\n                  \"OverlayTextColor\": \"Red\"\n                },\n                \"ResultVariable\": \"M2\"\n              },\n              {\n                \"Algorithm\": \"Math\",\n                \"MathExpression\": \"M2-M1\",\n                \"ResultVariable\": \"M3\"\n              }\n            ],\n            \"CalibrationCoefficients\": [\n              13,\n              8.7,\n              67.9\n            ],\n            \"UserCorrectionLinearityCoeff\": 45,\n            \"UserCorrectionBiasCoeff\": 56,\n            \"comment_LSL\": \"//Lower Specification Limit//\",\n            \"LSL\": 13.5,\n            \"comment_USL\": \"//Upper Specification Limit//\",\n            \"USL\": 15,\n            \"comment_LCL\": \"//Lower Control Limit//\",\n            \"LCL\": 13.5,\n            \"comment_UCL\": \"//Upper Control Limit//\",\n            \"UCL\": 15,\n            \"comment_ControlLimitsViolationThreshold\": \"//If 3 measurement results out of 1000, are crossing LCL and UCL then fail is detected//\",\n            \"ControlLimitsViolationThreshold\": [\n              3,\n              1000\n            ],\n            \"comment_SpecificationLimitsViolationThreshold\": \"//If 5 measurement results out of 5000, are crossing LSL and USL then fail is detected//\",\n            \"SpecificationLimitViolationThreshold\": [\n              5,\n              5000\n            ],\n            \"comment_Overlay\": \"//OverlayOptions contain Text, Co ordinates, Angle in Degrees, Text Size and Text Color for Overlay//\",\n            \"OverlayOptions\": {\n              \"OverlayEnable\": true,\n              \"OverlayText\": \"Collar Width\",\n              \"OverlayCoords\": [\n                5,\n                8\n              ],\n              \"OverlayAngle\": 56,\n              \"OverlayTextSize\": 6,\n              \"OverlayTextColor\": \"Red\"\n            },\n            \"DatalogEnable\": true,\n            \"DisplayIcon\": \"C:\\\\Desktop\\\\displayimage.png\"\n          }\n        ]\n      }\n    ]\n  },\n  \"AlgoParameters\": {\n    \"comment_RefROIEdgeOptions\": \"Reference ROI Edge Options is cluster of Edge Polarity, Kernel Size, Width, Minimum Edge Strength, Interpolation Type and Data Processing Method\",\n    \"RefROIEdgeOptions\": [\n      0,\n      2,\n      3,\n      3,\n      50,\n      0\n    ],\n    \"comment_RefROILineOptions\": \"Reference ROI Line Options is cluster of Number of lines, Type, Min. score, Max Score Orientation, Angle Range, Angle Tolerance, Step size, Min. SNR(db), Min Points (%) and Hough Iterations\",\n    \"RefROILineOptions\": [\n      1,\n      1,\n      10,\n      1000,\n      0,\n      10,\n      1,\n      10,\n      0,\n      25\n    ],\n    \"StepSize\": 14\n  }\n}") -> (0 "error out":errorcluster, 3 "VClusterOut":variant)   [LabVIEW 2015]
doc: "The input array of strings represent the <b>JSON paths</b> to specific elements in the JSON string. These elements are accessed through the path input and the output is provided in the form of <b>VCluster</b> (the bundled form of the input path elements). \nFurthermore, you may use the <b>Variant to Data</b> SubVI to convert back the Variant to the required Cluster type you want."
uses:
  <vilib>/Utility/Data Type/Type Definitions/Data Type.ctl
  <vilib>/regexp/Match Regular Expression.xnode
  <vilib>/addons/_JKI.lib/Serialization/JSON/JKI JSON Serialization.lvlib
  <vilib>/Utility/Data Type/NI_Data Type.lvlib
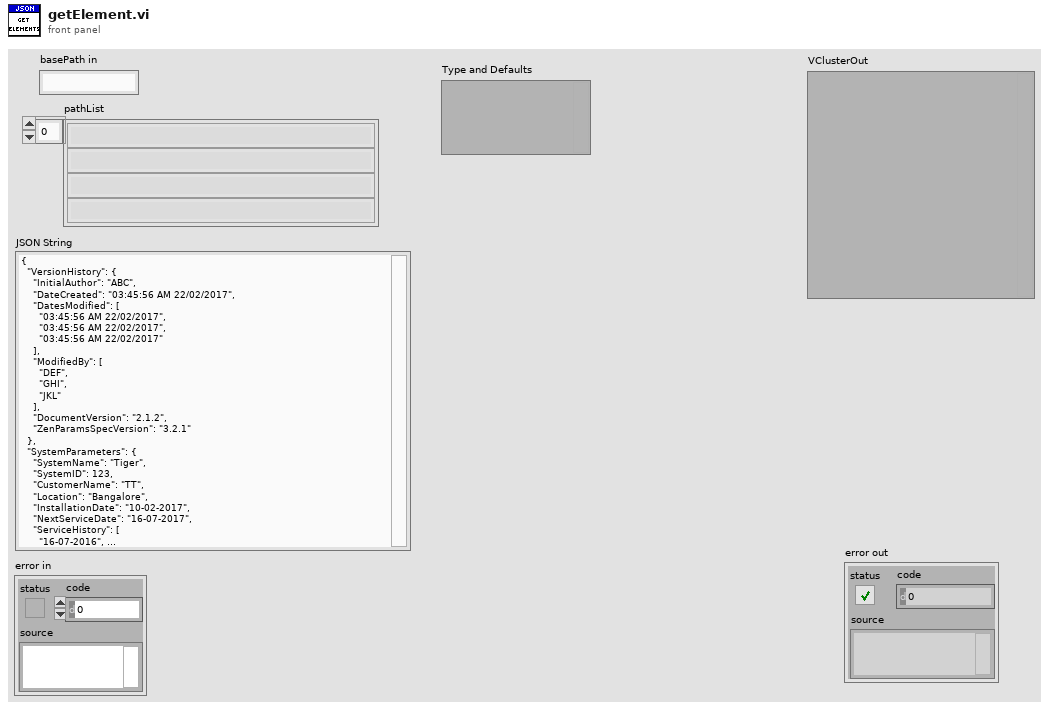
[diagram p1: front panel]
types:
  T1 = typedef "NI_Data Type.lvlib/Data Type.ctl" = enum8{"Invalid Type", "Void", "I8", "I16", "I32", "I64", "U8", "U16", "U32", "U64", "Single Float", "Double Float", "Extended Float", "Single Complex", "Double Complex", "Extended Complex", "Enum U8", "Enum U16", "Enum U32", "Enum U64", "Single Float With Unit", "Double Float With Unit", "Extended Float With Unit", "Single Complex with Unit", "Double Complex with Unit", "Extended Complex with Unit", "Boolean", "String", "Path", "Picture", "Tag", "Array", "Cluster", "Variant", "LV Variant", "Waveform", "Timestamp", "Digital Waveform", "Digital Data", "ExpressData", "Refnum", "External Data", "VI", "Poly VI", "LabVIEW Class Instance", "Fixed Point"}
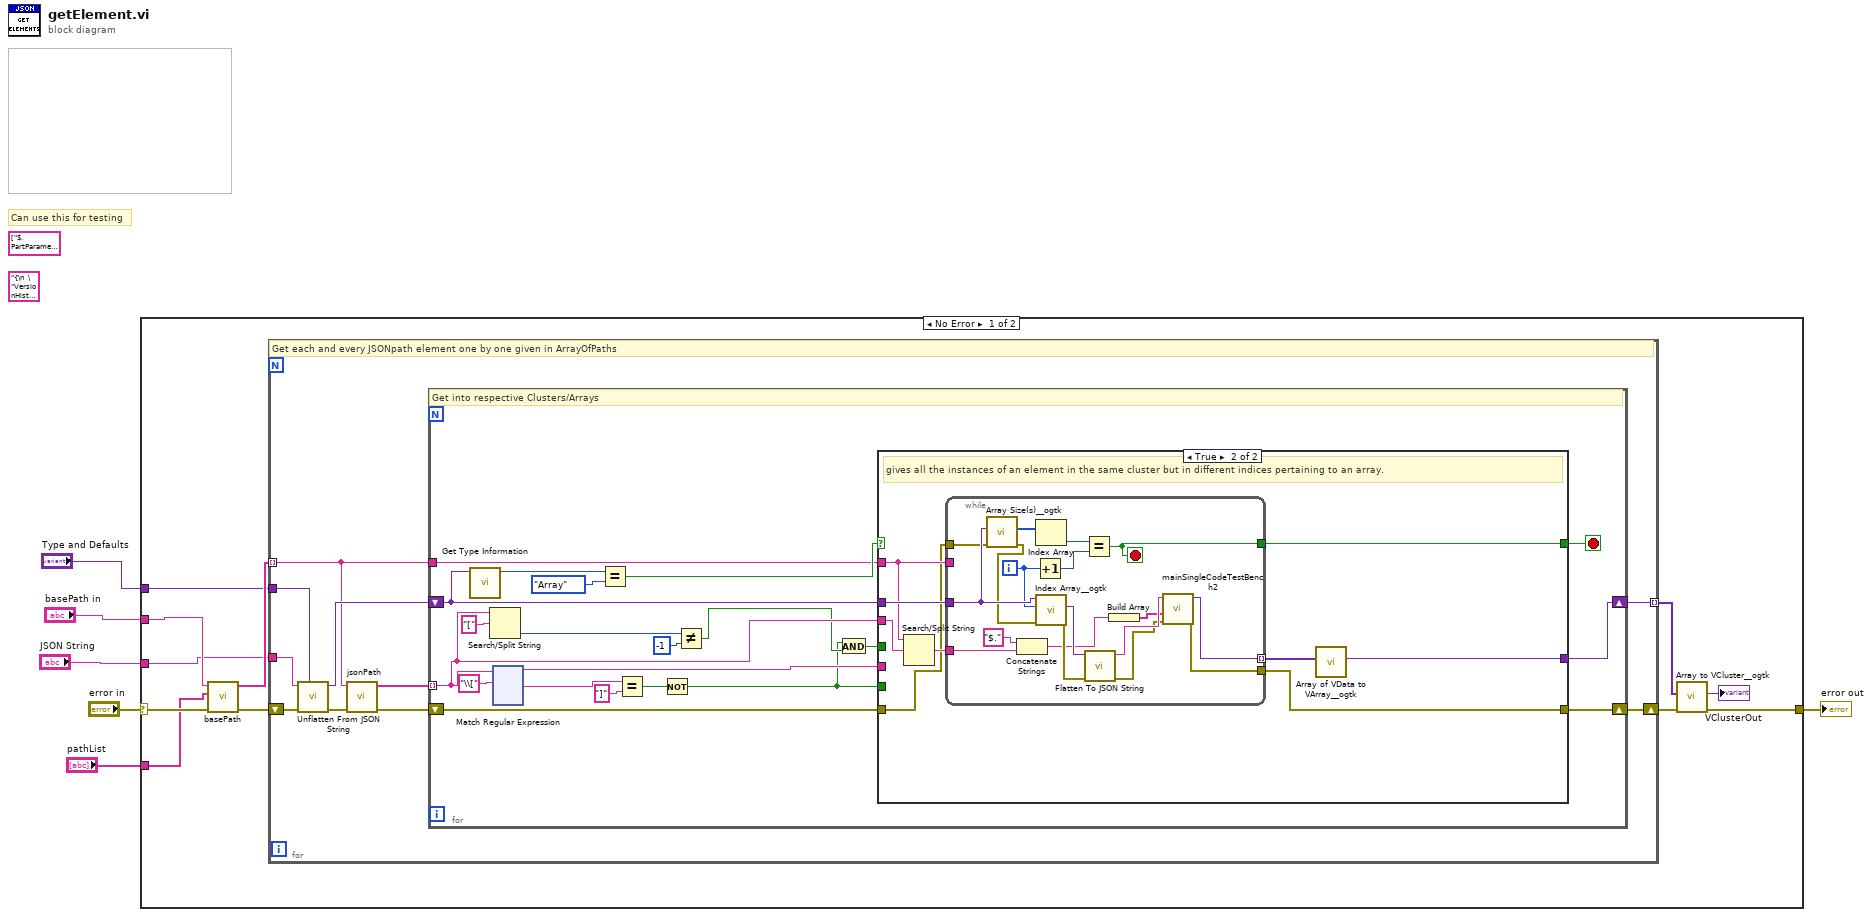
[diagram p0: block diagram]
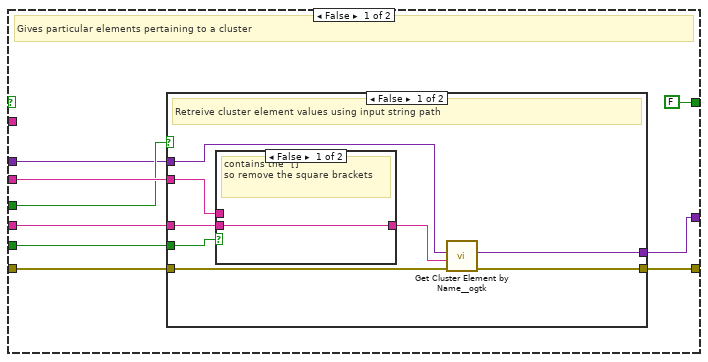
[diagram p2: hidden frame]
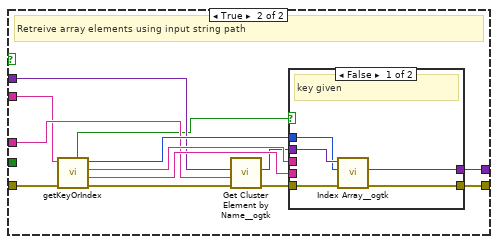
[diagram p4: hidden frame]
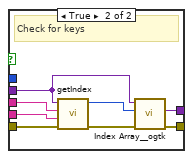
[diagram p5: hidden frame]
diagram:
  (unwired) string[] ["$.PartParameters.PartsList[Name=ECU1512]"] ("ArrayOfPaths")
  (unwired) "{\n  \"VersionHistory\": {\n    \"InitialAuthor\": \"ABC\",\n    \"DateCreated\": \"03:45:56 AM 22/02/2017\",\n    \"DatesModified\": [\n      \"03:45:56 AM 22/02/2017\",\n      \"03:45:56 AM 22/02/2017\",\n      \"03:45:56 AM 22/02/2017\"\n    ],\n    \"ModifiedBy\": [\n      \"DEF\",\n      \"GHI\",\n      \"JKL\"\n    ],\n    \"DocumentVersion\": \"2.1.2\",\n    \"ZenParamsSpecVersion\": \"3.2.1\"\n  },\n  \"SystemParameters\": {\n    \"SystemName\": \"Tiger\",\n    \"SystemID\": 123,\n    \"CustomerName\": \"TT\",\n    \"Location\": \"Bangalore\",\n    \"InstallationDate\": \"10-02-2017\",\n    \"NextServiceDate\": \"16-07-2017\",\n    \"ServiceHistory\": [\n      \"16-07-2016\",\n      \"16-08-2016\"\n    ],\n    \"CompatibleZenGage\": \"1.1\",\n    \"TotalNumberOfCameras\": 3,\n    \"NumberOfRacks\": 1,\n    \"SoftwareFeature\": {\n      \"comment_SoftwareFeatures\": \"//Software feature contains controls to Enable/Disable POST, Cp Cpk Report, Analytics, Data Logging and control to set value for Maximum Digital Zoom//\",\n      \"POSTEnable\": true,\n      \"CpCpkReportEnable\": true,\n      \"AnalyticsEnable\": true,\n      \"DataLoggingEnable\": true,\n      \"MaxDigitalZoom\": 5\n    },\n    \"GuideHorizontalPositioningEnable\": true,\n    \"comment_Sensor\": \"//Sensor section contains Name, Unique Id, Controller IO number and Triggering Edge of each sensor//\",\n    \"Sensor\": [\n      {\n        \"Name\": \"pqr\",\n        \"Id\": 1,\n        \"ControllerIONumber\": 12,\n        \"Edge\": \"FALLING\"\n      },\n      {\n        \"Name\": \"stu\",\n        \"Id\": 2,\n        \"ControllerIONumber\": 12,\n        \"Edge\": \"FALLING\"\n      },\n      {\n        \"Name\": \"vwx\",\n        \"Id\": 3,\n        \"ControllerIONumber\": 12,\n        \"Edge\": \"FALLING\"\n      }\n    ],\n    \"comment_Light\": \"//Light section contains Name, Unique Id, Type (Can be Bright field, Dark field, Back light, Front light, Diffuse light, Co-Axial diffuse etc.), Controller IO number and Level (HIGH or LOW) of each Light//\",\n    \"Light\": [\n      {\n        \"Name\": \"Light1\",\n        \"Id\": 1,\n        \"Type\": \"Back\",\n        \"ControllerIONumber\": 23,\n        \"Level\": \"HIGH\"\n      },\n      {\n        \"Name\": \"Light2\",\n        \"Id\": 2,\n        \"Type\": \"Front\",\n        \"ControllerIONumber\": 23,\n        \"Level\": \"HIGH\"\n      },\n      {\n        \"Name\": \"Light3\",\n        \"Id\": 3,\n        \"Type\": \"Back\",\n        \"ControllerIONumber\": 23,\n        \"Level\": \"HIGH\"\n      }\n    ],\n    \"comment_Camera\": \"//Camera section contains Camera Id, Type (Top, Side or Front), Model, Area of Interest (AOI), Trigger Mode, Controller IO Number, Triggering Edge, Pulse Width, Exposure Time in micro seconds, Interface Type (Allowed values are USB3, GigE, USB2), Gain in dB, Calibration details (Date and file path) of each camera//\",\n    \"Camera\": [\n      {\n        \"Id\": 1,\n        \"Type\": \"Top\",\n        \"Model\": \"Basler Ace 5MP\",\n        \"AOI\": [\n          12,\n          34,\n          56,\n          78\n        ],\n        \"TriggerMode\": \"External\",\n        \"ControllerIONumber\": 34,\n        \"Edge\": \"FALLING\",\n        \"PulseWidth\": 233,\n        \"ExposureTimeUSec\": 12,\n        \"InterfaceType\": \"USB3\",\n        \"GainIndB\": 6,\n        \"CalibrationDate\": \"12-01-2017\",\n        \"CalibrationFilePath\": \"C:\\\\Users\\\\veenaj\\\\Desktop\"\n      },\n      {\n        \"Id\": 2,\n        \"Type\": \"Side\",\n        \"Model\": \"Basler Ace 5MP\",\n        \"AOI\": [\n          12,\n          34,\n          56,\n          78\n        ],\n        \"TriggerMode\": \"External\",\n        \"ControllerIONumber\": 34,\n        \"Edge\": \"FALLING\",\n        \"PulseWidth\": 233,\n        \"ExposureTimeUSec\": 12,\n        \"InterfaceType\": \"USB3\",\n        \"GainIndB\": 6,\n        \"CalibrationDate\": \"12/04/17\",\n        \"CalibrationFilePath\": \"C:\\\\Desktop\\\\Calibration\"\n      },\n      {\n        \"Id\": 3,\n        \"Type\": \"Front\",\n        \"Model\": \"Basler Ace 5MP\",\n        \"AOI\": [\n          12,\n          34,\n          56,\n          78\n        ],\n        \"TriggerMode\": \"External\",\n        \"ControllerIONumber\": 34,\n        \"Edge\": \"FALLING\",\n        \"PulseWidth\": 233,\n        \"ExposureTimeUSec\": 12,\n        \"InterfaceType\": \"USB3\",\n        \"GainIndB\": 6,\n        \"CalibrationDate\": \"12/04/17\",\n        \"CalibrationFilePath\": \"C:\\\\Desktop\\\\Calibration\"\n      }\n    ]\n  },\n  \"PartParameters\": {\n    \"comment_PartParameters\": \"//Parts Parameters section includes Number of Parts configured and Parts List. Part List contains Name, Parallel Trigger Threads, Number of measurements and Measurement details//\",\n    \"NumberOfPartsConfigured\": 2,\n    \"PartsList\": [\n      {\n        \"Name\": \"ECU1511\",\n        \"comment_ParallelTriggerThreads\": \"//ParallelTriggerThreads contain Thread Name, Thread Id and Imaging Views. Combination of Camera and Light(s) is defined in Imaging View along with Sensor to Light Delay (in micro seconds), Light to Camera Trigger Delay, Light Pulse Width and Reference Co-ordinate system. Each Imaging View is given a Name and unique ImageId. Camera and Light(s) are accessed by their unique Ids.//\",\n        \"ParallelTriggerThreads\": [\n          {\n            \"ThreadName\": \"TopRack\",\n            \"ThreadId\": 1,\n            \"ImagingViews\": [\n              {\n                \"ImageId\": 1,\n                \"ViewName\": \"TopProfileView\",\n                \"CameraId\": 3,\n                \"LightIds\": [\n                  1,\n                  4,\n                  5\n                ],\n                \"SensorToLightDelayinUSec\": 12,\n                \"LightToCameraTriggerDelay\": 24,\n                \"LightPulseWidth\": 123,\n                \"ReferenceCoordSystem\": {\n                  \"Method\": [\n                    \"A\",\n                    \"B\",\n                    \"C\",\n                    \"D\",\n                    \"R\",\n                    \"V\"\n                  ],\n                  \"comment_RefROI\": \"//Reference ROI is cluster of Left, Top, Right, Bottom and Rotation values//\",\n                  \"ROI1\": [\n                    1014,\n                    95,\n                    1290,\n                    520,\n                    0\n                  ],\n                  \"ROI2\": [\n                    740,\n                    70,\n                    1040,\n                    340,\n                    0\n                  ],\n                  \"ROI3\": [\n                    1060,\n                    88,\n                    723,\n                    85,\n                    0\n                  ],\n                  \"Name\": \"FirstReference\"\n                }\n              },\n              {\n                \"ImageId\": 2,\n                \"ViewName\": \"TopLightView\",\n                \"CameraId\": 2,\n                \"LightIds\": [\n                  2,\n                  3,\n                  5\n                ],\n                \"SensorToLightDelayinUSec\": 12,\n                \"LightToCameraTriggerDelay\": 24,\n                \"LightPulseWidth\": 123,\n                \"ReferenceCoordSystem\": {\n                  \"Method\": [\n                    \"A\",\n                    \"B\",\n                    \"C\",\n                    \"D\",\n                    \"R\",\n                    \"V\"\n                  ],\n                  \"comment_RefROI\": \"//Reference ROI is cluster of Left, Top, Right, Bottom and Rotation values//\",\n                  \"ROI1\": [\n                    1014,\n                    95,\n                    1290,\n                    520,\n                    0\n                  ],\n                  \"ROI2\": [\n                    740,\n                    70,\n                    1040,\n                    340,\n                    0\n                  ],\n                  \"ROI3\": [\n                    1060,\n                    88,\n                    723,\n                    85,\n                    0\n                  ],\n                  \"Name\": \"FirstReference\"\n                }\n              }\n            ]\n          },\n          {\n            \"ThreadName\": \"BottomRack\",\n            \"ThreadId\": 2,\n            \"ImagingViews\": [\n              {\n                \"ImageId\": 1,\n                \"ViewName\": \"TopProfileView\",\n                \"CameraId\": 3,\n                \"LightIds\": [\n                  1,\n                  4,\n                  5\n                ],\n                \"SensorToLightDelayinUSec\": 12,\n                \"LightToCameraTriggerDelay\": 24,\n                \"LightPulseWidth\": 123,\n                \"ReferenceCoordSystem\": {\n                  \"Method\": [\n                    \"A\",\n                    \"B\",\n                    \"C\",\n                    \"D\",\n                    \"R\",\n                    \"V\"\n                  ],\n                  \"comment_RefROI\": \"//Reference ROI is cluster of Left, Top, Right, Bottom and Rotation values//\",\n                  \"ROI1\": [\n                    1014,\n                    95,\n                    1290,\n                    520,\n                    0\n                  ],\n                  \"ROI2\": [\n                    740,\n                    70,\n                    1040,\n                    340,\n                    0\n                  ],\n                  \"ROI3\": [\n                    1060,\n                    88,\n                    723,\n                    85,\n                    0\n                  ],\n                  \"Name\": \"FirstReference\"\n                }\n              },\n              {\n                \"ImageId\": 2,\n                \"ViewName\": \"TopLightView\",\n                \"CameraId\": 2,\n                \"LightIds\": [\n                  2,\n                  3,\n                  5\n                ],\n                \"SensorToLightDelayinUSec\": 12,\n                \"LightToCameraTriggerDelay\": 24,\n                \"LightPulseWidth\": 123,\n                \"ReferenceCoordSystem\": {\n                  \"Method\": [\n                    \"A\",\n                    \"B\",\n                    \"C\",\n                    \"D\",\n                    \"R\",\n                    \"V\"\n                  ],\n                  \"comment_RefROI\": \"//Reference ROI is cluster of Left, Top, Right, Bottom and Rotation values//\",\n                  \"ROI1\": [\n                    1014,\n                    95,\n                    1290,\n                    520,\n                    0\n                  ],\n                  \"ROI2\": [\n                    740,\n                    70,\n                    1040,\n                    340,\n                    0\n                  ],\n                  \"ROI3\": [\n                    1060,\n                    88,\n                    723,\n                    85,\n                    0\n                  ],\n                  \"Name\": \"FirstReference\"\n                }\n              }\n            ]\n          },\n          {\n            \"ThreadName\": \"DentIdentification\",\n            \"ThreadId\": 3,\n            \"ImagingViews\": [\n              {\n                \"ImageId\": 1,\n                \"ViewName\": \"TopProfileView\",\n                \"CameraId\": 3,\n                \"LightIds\": [\n                  1,\n                  4,\n                  5\n                ],\n                \"SensorToLightDelayinUSec\": 12,\n                \"LightToCameraTriggerDelay\": 24,\n                \"LightPulseWidth\": 123,\n                \"ReferenceCoordSystem\": {\n                  \"Method\": [\n                    \"A\",\n                    \"B\",\n                    \"C\",\n                    \"D\",\n                    \"R\",\n                    \"V\"\n                  ],\n                  \"comment_RefROI\": \"//Reference ROI is cluster of Left, Top, Right, Bottom and Rotation values//\",\n                  \"ROI1\": [\n                    23,\n                    78,\n                    99,\n                    25,\n                    0\n                  ],\n                  \"ROI2\": [\n                    67,\n                    97,\n                    43,\n                    9,\n                    0\n                  ],\n                  \"ROI3\": [\n                    45,\n                    88,\n                    723,\n                    85,\n                    0\n                  ],\n                  \"Name\": \"FirstReference\"\n                }\n              }\n            ]\n          }\n        ],\n        \"Number of Measurements\": 3,\n        \"comment_Measurements\": \"//Measurements section contains Name, Type, Enable, Algorithm Sequence, Calibration Co-efficients, User Correction Linearity Coefficients, User Correction Bias Coefficients, LSL, USL, LCL, UCL, Control Limits Violation Threshold, Specification Limits Violation Threshold, Overlay Options, Datalog Enable, Display Icon path for each Measurement//\",\n        \"Measurements\": [\n          {\n            \"Name\": \"CollarWidth\",\n            \"comment_Type\": \"//Type can be Linear or Angle//\",\n            \"Type\": \"Linear\",\n            \"Enable\": true,\n            \"comment_AlgorithmSequence\": \"//Particular Measurement may require sequence of Algorithms. ThreadId and ThreadImageId are mentioned in each Algorithm which corresponds to particular combination of Camera and Light Ids. Result of each Algorithm is stored in a variable and final result is calculated using Math Expression defined.//\",\n            \"AlgorithmSequence\": [\n              {\n                \"AlgoName\": \"MaxClamp\",\n                \"ThreadId\": 1,\n                \"ThreadImageId\": 2,\n                \"Option1\": \"\",\n                \"Option2\": \"\",\n                \"Option3\": \"\",\n                \"LocalRef\": {\n                  \"LocalCoordinateSystemEnable\": true,\n                  \"Method\": [\n                    \"A\",\n                    \"B\",\n                    \"C\",\n                    \"D\",\n                    \"R\",\n                    \"V\"\n                  ],\n                  \"comment_LocalRefROI\": \"//Local Reference ROI is cluster of Left, Top, Right, Bottom and Rotation values//\",\n                  \"ROIs\": [\n                    [\n                      23,\n                      78,\n                      99,\n                      25,\n                      0\n                    ],\n                    [\n                      67,\n                      97,\n                      43,\n                      9,\n                      0\n                    ],\n                    [\n                      45,\n                      88,\n                      723,\n                      85,\n                      0\n                    ]\n                  ],\n                  \"Name\": \"CollarWidthLocalReference\"\n                },\n                \"LocalROIs\": [\n                  [\n                    23,\n                    78,\n                    99,\n                    25,\n                    0\n                  ],\n                  [\n                    67,\n                    97,\n                    43,\n                    9,\n                    0\n                  ],\n                  [\n                    45,\n                    88,\n                    723,\n                    85,\n                    0\n                  ]\n                ],\n                \"comment_Overlay\": \"//OverlayOptions contain Text, Co ordinates, Angle in Degrees, Text Size and Text Color for Overlay//\",\n                \"OverlayOptions\": {\n                  \"OverlayEnable\": true,\n                  \"OverlayText\": \"Collar Width\",\n                  \"OverlayCoords\": [\n                    5,\n                    8\n                  ],\n                  \"OverlayAngle\": 56,\n                  \"OverlayTextSize\": 6,\n                  \"OverlayTextColor\": \"Red\"\n                },\n                \"ResultVariable\": \"M1\"\n              },\n              {\n                \"AlgoName\": \"MoveXYTable\",\n                \"XYDelta\": [\n                  56,\n                  -33.8\n                ]\n              },\n              {\n                \"AlgoName\": \"MaxClamp\",\n                \"ThreadId\": 1,\n                \"ThreadImageId\": 2,\n                \"Option1\": \"\",\n                \"Option2\": \"\",\n                \"Option3\": \"\",\n                \"LocalRef\": {\n                  \"LocalCoordinateSystemEnable\": true,\n                  \"Method\": [\n                    \"A\",\n                    \"B\",\n                    \"C\",\n                    \"D\",\n                    \"R\",\n                    \"V\"\n                  ],\n                  \"ROIs\": [\n                    [\n                      23,\n                      78,\n                      99,\n                      25,\n                      0\n                    ],\n                    [\n                      67,\n                      97,\n                      43,\n                      9,\n                      0\n                    ],\n                    [\n                      45,\n                      88,\n                      723,\n                      85,\n                      0\n                    ]\n                  ],\n                  \"Name\": \"CollarWidthLocalReference\"\n                },\n                \"LocalROIs\": [\n                  [\n                    23,\n                    78,\n                    99,\n                    25,\n                    0\n                  ],\n                  [\n                    67,\n                    97,\n                    43,\n                    9,\n                    0\n                  ],\n                  [\n                    45,\n                    88,\n                    723,\n                    85,\n                    0\n                  ]\n                ],\n                \"comment_Overlay\": \"//OverlayOptions contain Text, Co ordinates, Angle in Degrees, Text Size and Text Color for Overlay//\",\n                \"OverlayOptions\": {\n                  \"OverlayEnable\": true,\n                  \"OverlayText\": \"Collar Width\",\n                  \"OverlayCoords\": [\n                    5,\n                    8\n                  ],\n                  \"OverlayAngle\": 56,\n                  \"OverlayTextSize\": 6,\n                  \"OverlayTextColor\": \"Red\"\n                },\n                \"ResultVariable\": \"M2\"\n              },\n              {\n                \"Algorithm\": \"Math\",\n                \"MathExpression\": \"M2-M1\",\n                \"ResultVariable\": \"M3\"\n              }\n            ],\n            \"CalibrationCoefficients\": [\n              13,\n              8.7,\n              67.9\n            ],\n            \"UserCorrectionLinearityCoeff\": 45,\n            \"UserCorrectionBiasCoeff\": 56,\n            \"comment_LSL\": \"//Lower Specification Limit//\",\n            \"LSL\": 13.5,\n            \"comment_USL\": \"//Upper Specification Limit//\",\n            \"USL\": 15,\n            \"comment_LCL\": \"//Lower Control Limit//\",\n            \"LCL\": 13.5,\n            \"comment_UCL\": \"//Upper Control Limit//\",\n            \"UCL\": 15,\n            \"comment_ControlLimitsViolationThreshold\": \"//If 3 measurement results out of 1000, are crossing LCL and UCL then fail is detected//\",\n            \"ControlLimitsViolationThreshold\": [\n              3,\n              1000\n            ],\n            \"comment_SpecificationLimitsViolationThreshold\": \"//If 5 measurement results out of 5000, are crossing LSL and USL then fail is detected//\",\n            \"SpecificationLimitViolationThreshold\": [\n              5,\n              5000\n            ],\n            \"comment_Overlay\": \"//OverlayOptions contain Text, Co ordinates, Angle in Degrees, Text Size and Text Color for Overlay//\",\n            \"OverlayOptions\": {\n              \"OverlayEnable\": true,\n              \"OverlayText\": \"Collar Width\",\n              \"OverlayCoords\": [\n                5,\n                8\n              ],\n              \"OverlayAngle\": 56,\n              \"OverlayTextSize\": 6,\n              \"OverlayTextColor\": \"Red\"\n            },\n            \"DatalogEnable\": true,\n            \"DisplayIcon\": \"C:\\\\Desktop\\\\displayimage.png\"\n          },\n          {\n            \"Name\": \"Length\",\n            \"comment_Type\": \"//Type can be Linear or Angle//\",\n            \"Type\": \"Linear\",\n            \"Enable\": true,\n            \"comment_AlgorithmSequence\": \"//Particular Measurement may require sequence of Algorithms. ThreadId and ThreadImageId are mentioned in each Algorithm which corresponds to particular combination of Camera and Light Ids. Result of each Algorithm is stored in a variable and final result is calculated using Math Expression defined.//\",\n            \"AlgorithmSequence\": [\n              {\n                \"AlgoName\": \"MaxClamp\",\n                \"ThreadId\": 1,\n                \"ThreadImageId\": 2,\n                \"Option1\": \"\",\n                \"Option2\": \"\",\n                \"Option3\": \"\",\n                \"LocalRef\": {\n                  \"LocalCoordinateSystemEnable\": true,\n                  \"Method\": [\n                    \"A\",\n                    \"B\",\n                    \"C\",\n                    \"D\",\n                    \"R\",\n                    \"V\"\n                  ],\n                  \"comment_LocalRefROI\": \"//Local Reference ROI is cluster of Left, Top, Right, Bottom and Rotation values//\",\n                  \"ROIs\": [\n                    [\n                      23,\n                      78,\n                      99,\n                      25,\n                      0\n                    ],\n                    [\n                      67,\n                      97,\n                      43,\n                      9,\n                      0\n                    ],\n                    [\n                      45,\n                      88,\n                      723,\n                      85,\n                      0\n                    ]\n                  ],\n                  \"Name\": \"CollarWidthLocalReference\"\n                },\n                \"LocalROIs\": [\n                  [\n                    23,\n                    78,\n                    99,\n                    25,\n                    0\n                  ],\n                  [\n                    67,\n                    97,\n                    43,\n                    9,\n                    0\n                  ],\n                  [\n                    45,\n                    88,\n                    723,\n                    85,\n                    0\n                  ]\n                ],\n                \"comment_Overlay\": \"//OverlayOptions contain Text, Co ordinates, Angle in Degrees, Text Size and Text Color for Overlay//\",\n                \"OverlayOptions\": {\n                  \"OverlayEnable\": true,\n                  \"OverlayText\": \"Collar Width\",\n                  \"OverlayCoords\": [\n                    5,\n                    8\n                  ],\n                  \"OverlayAngle\": 56,\n                  \"OverlayTextSize\": 6,\n                  \"OverlayTextColor\": \"Red\"\n                },\n                \"ResultVariable\": \"M1\"\n              },\n              {\n                \"AlgoName\": \"MoveXYTable\",\n                \"XYDelta\": [\n                  56,\n                  -33.8\n                ]\n              },\n              {\n                \"AlgoName\": \"MaxClamp\",\n                \"ThreadId\": 1,\n                \"ThreadImageId\": 2,\n                \"Option1\": \"\",\n                \"Option2\": \"\",\n                \"Option3\": \"\",\n                \"LocalRef\": {\n                  \"LocalCoordinateSystemEnable\": true,\n                  \"Method\": [\n                    \"A\",\n                    \"B\",\n                    \"C\",\n                    \"D\",\n                    \"R\",\n                    \"V\"\n                  ],\n                  \"ROIs\": [\n                    [\n                      23,\n                      78,\n                      99,\n                      25,\n                      0\n                    ],\n                    [\n                      67,\n                      97,\n                      43,\n                      9,\n                      0\n                    ],\n                    [\n                      45,\n                      88,\n                      723,\n                      85,\n                      0\n                    ]\n                  ],\n                  \"Name\": \"CollarWidthLocalReference\"\n                },\n                \"LocalROIs\": [\n                  [\n                    23,\n                    78,\n                    99,\n                    25,\n                    0\n                  ],\n                  [\n                    67,\n                    97,\n                    43,\n                    9,\n                    0\n                  ],\n                  [\n                    45,\n                    88,\n                    723,\n                    85,\n                    0\n                  ]\n                ],\n                \"comment_Overlay\": \"//OverlayOptions contain Text, Co ordinates, Angle in Degrees, Text Size and Text Color for Overlay//\",\n                \"OverlayOptions\": {\n                  \"OverlayEnable\": true,\n                  \"OverlayText\": \"Collar Width\",\n                  \"OverlayCoords\": [\n                    5,\n                    8\n                  ],\n                  \"OverlayAngle\": 56,\n                  \"OverlayTextSize\": 6,\n                  \"OverlayTextColor\": \"Red\"\n                },\n                \"ResultVariable\": \"M2\"\n              },\n              {\n                \"Algorithm\": \"Math\",\n                \"MathExpression\": \"M2-M1\",\n                \"ResultVariable\": \"M3\"\n              }\n            ],\n            \"CalibrationCoefficients\": [\n              13,\n              8.7,\n              67.9\n            ],\n            \"UserCorrectionLinearityCoeff\": 45,\n            \"UserCorrectionBiasCoeff\": 56,\n            \"comment_LSL\": \"//Lower Specification Limit//\",\n            \"LSL\": 13.5,\n            \"comment_USL\": \"//Upper Specification Limit//\",\n            \"USL\": 15,\n            \"comment_LCL\": \"//Lower Control Limit//\",\n            \"LCL\": 13.5,\n            \"comment_UCL\": \"//Upper Control Limit//\",\n            \"UCL\": 15,\n            \"comment_ControlLimitsViolationThreshold\": \"//If 3 measurement results out of 1000, are crossing LCL and UCL then fail is detected//\",\n            \"ControlLimitsViolationThreshold\": [\n              3,\n              1000\n            ],\n            \"comment_SpecificationLimitsViolationThreshold\": \"//If 5 measurement results out of 5000, are crossing LSL and USL then fail is detected//\",\n            \"SpecificationLimitViolationThreshold\": [\n              5,\n              5000\n            ],\n            \"comment_Overlay\": \"//OverlayOptions contain Text, Co ordinates, Angle in Degrees, Text Size and Text Color for Overlay//\",\n            \"OverlayOptions\": {\n              \"OverlayEnable\": true,\n              \"OverlayText\": \"Collar Width\",\n              \"OverlayCoords\": [\n                5,\n                8\n              ],\n              \"OverlayAngle\": 56,\n              \"OverlayTextSize\": 6,\n              \"OverlayTextColor\": \"Red\"\n            },\n            \"DatalogEnable\": true,\n            \"DisplayIcon\": \"C:\\\\Desktop\\\\displayimage.png\"\n          },\n          {\n            \"Name\": \"Length2\",\n            \"comment_Type\": \"//Type can be Linear or Angle//\",\n            \"Type\": \"Linear\",\n            \"Enable\": true,\n            \"comment_AlgorithmSequence\": \"//Particular Measurement may require sequence of Algorithms. ThreadId and ThreadImageId are mentioned in each Algorithm which corresponds to particular combination of Camera and Light Ids. Result of each Algorithm is stored in a variable and final result is calculated using Math Expression defined.//\",\n            \"AlgorithmSequence\": [\n              {\n                \"AlgoName\": \"MaxClamp\",\n                \"ThreadId\": 1,\n                \"ThreadImageId\": 2,\n                \"Option1\": \"\",\n                \"Option2\": \"\",\n                \"Option3\": \"\",\n                \"LocalRef\": {\n                  \"LocalCoordinateSystemEnable\": true,\n                  \"Method\": [\n                    \"A\",\n                    \"B\",\n                    \"C\",\n                    \"D\",\n                    \"R\",\n                    \"V\"\n                  ],\n                  \"comment_LocalRefROI\": \"//Local Reference ROI is cluster of Left, Top, Right, Bottom and Rotation values//\",\n                  \"ROIs\": [\n                    [\n                      23,\n                      78,\n                      99,\n                      25,\n                      0\n                    ],\n                    [\n                      67,\n                      97,\n                      43,\n                      9,\n                      0\n                    ],\n                    [\n                      45,\n                      88,\n                      723,\n                      85,\n                      0\n                    ]\n                  ],\n                  \"Name\": \"CollarWidthLocalReference\"\n                },\n                \"LocalROIs\": [\n                  [\n                    23,\n                    78,\n                    99,\n                    25,\n                    0\n                  ],\n                  [\n                    67,\n                    97,\n                    43,\n                    9,\n                    0\n                  ],\n                  [\n                    45,\n                    88,\n                    723,\n                    85,\n                    0\n                  ]\n                ],\n                \"comment_Overlay\": \"//OverlayOptions contain Text, Co ordinates, Angle in Degrees, Text Size and Text Color for Overlay//\",\n                \"OverlayOptions\": {\n                  \"OverlayEnable\": true,\n                  \"OverlayText\": \"Collar Width\",\n                  \"OverlayCoords\": [\n                    5,\n                    8\n                  ],\n                  \"OverlayAngle\": 56,\n                  \"OverlayTextSize\": 6,\n                  \"OverlayTextColor\": \"Red\"\n                },\n                \"ResultVariable\": \"M1\"\n              },\n              {\n                \"AlgoName\": \"MoveXYTable\",\n                \"XYDelta\": [\n                  56,\n                  -33.8\n                ]\n              },\n              {\n                \"AlgoName\": \"MaxClamp\",\n                \"ThreadId\": 1,\n                \"ThreadImageId\": 2,\n                \"Option1\": \"\",\n                \"Option2\": \"\",\n                \"Option3\": \"\",\n                \"LocalRef\": {\n                  \"LocalCoordinateSystemEnable\": true,\n                  \"Method\": [\n                    \"A\",\n                    \"B\",\n                    \"C\",\n                    \"D\",\n                    \"R\",\n                    \"V\"\n                  ],\n                  \"ROIs\": [\n                    [\n                      23,\n                      78,\n                      99,\n                      25,\n                      0\n                    ],\n                    [\n                      67,\n                      97,\n                      43,\n                      9,\n                      0\n                    ],\n                    [\n                      45,\n                      88,\n                      723,\n                      85,\n                      0\n                    ]\n                  ],\n                  \"Name\": \"CollarWidthLocalReference\"\n                },\n                \"LocalROIs\": [\n                  [\n                    23,\n                    78,\n                    99,\n                    25,\n                    0\n                  ],\n                  [\n                    67,\n                    97,\n                    43,\n                    9,\n                    0\n                  ],\n                  [\n                    45,\n                    88,\n                    723,\n                    85,\n                    0\n                  ]\n                ],\n                \"comment_Overlay\": \"//OverlayOptions contain Text, Co ordinates, Angle in Degrees, Text Size and Text Color for Overlay//\",\n                \"OverlayOptions\": {\n                  \"OverlayEnable\": true,\n                  \"OverlayText\": \"Collar Width\",\n                  \"OverlayCoords\": [\n                    5,\n                    8\n                  ],\n                  \"OverlayAngle\": 56,\n                  \"OverlayTextSize\": 6,\n                  \"OverlayTextColor\": \"Red\"\n                },\n                \"ResultVariable\": \"M2\"\n              },\n              {\n                \"Algorithm\": \"Math\",\n                \"MathExpression\": \"M2-M1\",\n                \"ResultVariable\": \"M3\"\n              }\n            ],\n            \"CalibrationCoefficients\": [\n              13,\n              8.7,\n              67.9\n            ],\n            \"UserCorrectionLinearityCoeff\": 45,\n            \"UserCorrectionBiasCoeff\": 56,\n            \"comment_LSL\": \"//Lower Specification Limit//\",\n            \"LSL\": 13.5,\n            \"comment_USL\": \"//Upper Specification Limit//\",\n            \"USL\": 15,\n            \"comment_LCL\": \"//Lower Control Limit//\",\n            \"LCL\": 13.5,\n            \"comment_UCL\": \"//Upper Control Limit//\",\n            \"UCL\": 15,\n            \"comment_ControlLimitsViolationThreshold\": \"//If 3 measurement results out of 1000, are crossing LCL and UCL then fail is detected//\",\n            \"ControlLimitsViolationThreshold\": [\n              3,\n              1000\n            ],\n            \"comment_SpecificationLimitsViolationThreshold\": \"//If 5 measurement results out of 5000, are crossing LSL and USL then fail is detected//\",\n            \"SpecificationLimitViolationThreshold\": [\n              5,\n              5000\n            ],\n            \"comment_Overlay\": \"//OverlayOptions contain Text, Co ordinates, Angle in Degrees, Text Size and Text Color for Overlay//\",\n            \"OverlayOptions\": {\n              \"OverlayEnable\": true,\n              \"OverlayText\": \"Collar Width\",\n              \"OverlayCoords\": [\n                5,\n                8\n              ],\n              \"OverlayAngle\": 56,\n              \"OverlayTextSize\": 6,\n              \"OverlayTextColor\": \"Red\"\n            },\n            \"DatalogEnable\": true,\n            \"DisplayIcon\": \"C:\\\\Desktop\\\\displayimage.png\"\n          }\n        ]\n      },\n      {\n        \"Name\": \"ECU1512\",\n        \"comment_ParallelTriggerThreads\": \"//ParallelTriggerThreads contain Thread Name, Thread Id and Imaging Views. Combination of Camera and Light(s) is defined in Imaging View along with Sensor to Light Delay (in micro seconds), Light to Camera Trigger Delay, Light Pulse Width and Reference Co-ordinate system. Each Imaging View is given a Name and unique ImageId. Camera and Light(s) are accessed by their unique Ids.//\",\n        \"ParallelTriggerThreads\": [\n          {\n            \"ThreadName\": \"TopRack\",\n            \"ThreadId\": 1,\n            \"ImagingViews\": [\n              {\n                \"ImageId\": 1,\n                \"ViewName\": \"TopProfileView\",\n                \"CameraId\": 3,\n                \"LightIds\": [\n                  1,\n                  4,\n                  5\n                ],\n                \"SensorToLightDelayinUSec\": 12,\n                \"LightToCameraTriggerDelay\": 24,\n                \"LightPulseWidth\": 123,\n                \"ReferenceCoordSystem\": {\n                  \"Method\": [\n                    \"A\",\n                    \"B\",\n                    \"C\",\n                    \"D\",\n                    \"R\",\n                    \"V\"\n                  ],\n                  \"comment_RefROI\": \"//Reference ROI is cluster of Left, Top, Right, Bottom and Rotation values//\",\n                  \"ROI1\": [\n                    1014,\n                    95,\n                    1290,\n                    520,\n                    0\n                  ],\n                  \"ROI2\": [\n                    740,\n                    70,\n                    1040,\n                    340,\n                    0\n                  ],\n                  \"ROI3\": [\n                    1060,\n                    88,\n                    723,\n                    85,\n                    0\n                  ],\n                  \"Name\": \"FirstReference\"\n                }\n              },\n              {\n                \"ImageId\": 2,\n                \"ViewName\": \"TopLightView\",\n                \"CameraId\": 2,\n                \"LightIds\": [\n                  2,\n                  3,\n                  5\n                ],\n                \"SensorToLightDelayinUSec\": 12,\n                \"LightToCameraTriggerDelay\": 24,\n                \"LightPulseWidth\": 123,\n                \"ReferenceCoordSystem\": {\n                  \"Method\": [\n                    \"A\",\n                    \"B\",\n                    \"C\",\n                    \"D\",\n                    \"R\",\n                    \"V\"\n                  ],\n                  \"comment_RefROI\": \"//Reference ROI is cluster of Left, Top, Right, Bottom and Rotation values//\",\n                  \"ROI1\": [\n                    1014,\n                    95,\n                    1290,\n                    520,\n                    0\n                  ],\n                  \"ROI2\": [\n                    740,\n                    70,\n                    1040,\n                    340,\n                    0\n                  ],\n                  \"ROI3\": [\n                    1060,\n                    88,\n                    723,\n                    85,\n                    0\n                  ],\n                  \"Name\": \"FirstReference\"\n                }\n              }\n            ]\n          },\n          {\n            \"ThreadName\": \"BottomRack\",\n            \"ThreadId\": 2,\n            \"ImagingViews\": [\n              {\n                \"ImageId\": 1,\n                \"ViewName\": \"TopProfileView\",\n                \"CameraId\": 3,\n                \"LightIds\": [\n                  1,\n                  4,\n                  5\n                ],\n                \"SensorToLightDelayinUSec\": 12,\n                \"LightToCameraTriggerDelay\": 24,\n                \"LightPulseWidth\": 123,\n                \"ReferenceCoordSystem\": {\n                  \"Method\": [\n                    \"A\",\n                    \"B\",\n                    \"C\",\n                    \"D\",\n                    \"R\",\n                    \"V\"\n                  ],\n                  \"comment_RefROI\": \"//Reference ROI is cluster of Left, Top, Right, Bottom and Rotation values//\",\n                  \"ROI1\": [\n                    1014,\n                    95,\n                    1290,\n                    520,\n                    0\n                  ],\n                  \"ROI2\": [\n                    740,\n                    70,\n                    1040,\n                    340,\n                    0\n                  ],\n                  \"ROI3\": [\n                    1060,\n                    88,\n                    723,\n                    85,\n                    0\n                  ],\n                  \"Name\": \"FirstReference\"\n                }\n              },\n              {\n                \"ImageId\": 2,\n                \"ViewName\": \"TopLightView\",\n                \"CameraId\": 2,\n                \"LightIds\": [\n                  2,\n                  3,\n                  5\n                ],\n                \"SensorToLightDelayinUSec\": 12,\n                \"LightToCameraTriggerDelay\": 24,\n                \"LightPulseWidth\": 123,\n                \"ReferenceCoordSystem\": {\n                  \"Method\": [\n                    \"A\",\n                    \"B\",\n                    \"C\",\n                    \"D\",\n                    \"R\",\n                    \"V\"\n                  ],\n                  \"comment_RefROI\": \"//Reference ROI is cluster of Left, Top, Right, Bottom and Rotation values//\",\n                  \"ROI1\": [\n                    1014,\n                    95,\n                    1290,\n                    520,\n                    0\n                  ],\n                  \"ROI2\": [\n                    740,\n                    70,\n                    1040,\n                    340,\n                    0\n                  ],\n                  \"ROI3\": [\n                    1060,\n                    88,\n                    723,\n                    85,\n                    0\n                  ],\n                  \"Name\": \"FirstReference\"\n                }\n              }\n            ]\n          },\n          {\n            \"ThreadName\": \"DentIdentification\",\n            \"ThreadId\": 3,\n            \"ImagingViews\": [\n              {\n                \"ImageId\": 1,\n                \"ViewName\": \"TopProfileView\",\n                \"CameraId\": 3,\n                \"LightIds\": [\n                  1,\n                  4,\n                  5\n                ],\n                \"SensorToLightDelayinUSec\": 12,\n                \"LightToCameraTriggerDelay\": 24,\n                \"LightPulseWidth\": 123,\n                \"ReferenceCoordSystem\": {\n                  \"Method\": [\n                    \"A\",\n                    \"B\",\n                    \"C\",\n                    \"D\",\n                    \"R\",\n                    \"V\"\n                  ],\n                  \"comment_RefROI\": \"//Reference ROI is cluster of Left, Top, Right, Bottom and Rotation values//\",\n                  \"ROI1\": [\n                    23,\n                    78,\n                    99,\n                    25,\n                    0\n                  ],\n                  \"ROI2\": [\n                    67,\n                    97,\n                    43,\n                    9,\n                    0\n                  ],\n                  \"ROI3\": [\n                    45,\n                    88,\n                    723,\n                    85,\n                    0\n                  ],\n                  \"Name\": \"FirstReference\"\n                }\n              }\n            ]\n          }\n        ],\n        \"comment_Measurements\": \"//Measurements section contains Name, Type, Enable, Algorithm Sequence, Calibration Co-efficients, User Correction Linearity Coefficients, User Correction Bias Coefficients, LSL, USL, LCL, UCL, Control Limits Violation Threshold, Specification Limits Violation Threshold, Overlay Options, Datalog Enable, Display Icon path for each Measurement//\",\n        \"Measurements\": [\n          {\n            \"Name\": \"CollarWidth\",\n            \"comment_Type\": \"//Type can be Linear or Angle//\",\n            \"Type\": \"Linear\",\n            \"Enable\": true,\n            \"comment_AlgorithmSequence\": \"//Particular Measurement may require sequence of Algorithms. ThreadId and ThreadImageId are mentioned in each Algorithm which corresponds to particular combination of Camera and Light Ids. Result of each Algorithm is stored in a variable and final result is calculated using Math Expression defined.//\",\n            \"AlgorithmSequence\": [\n              {\n                \"AlgoName\": \"MaxClamp\",\n                \"ThreadId\": 1,\n                \"ThreadImageId\": 2,\n                \"Option1\": \"\",\n                \"Option2\": \"\",\n                \"Option3\": \"\",\n                \"LocalRef\": {\n                  \"LocalCoordinateSystemEnable\": true,\n                  \"Method\": [\n                    \"A\",\n                    \"B\",\n                    \"C\",\n                    \"D\",\n                    \"R\",\n                    \"V\"\n                  ],\n                  \"comment_LocalRefROI\": \"//Local Reference ROI is cluster of Left, Top, Right, Bottom and Rotation values//\",\n                  \"ROIs\": [\n                    [\n                      23,\n                      78,\n                      99,\n                      25,\n                      0\n                    ],\n                    [\n                      67,\n                      97,\n                      43,\n                      9,\n                      0\n                    ],\n                    [\n                      45,\n                      88,\n                      723,\n                      85,\n                      0\n                    ]\n                  ],\n                  \"Name\": \"CollarWidthLocalReference\"\n                },\n                \"LocalROIs\": [\n                  [\n                    23,\n                    78,\n                    99,\n                    25,\n                    0\n                  ],\n                  [\n                    67,\n                    97,\n                    43,\n                    9,\n                    0\n                  ],\n                  [\n                    45,\n                    88,\n                    723,\n                    85,\n                    0\n                  ]\n                ],\n                \"comment_Overlay\": \"//OverlayOptions contain Text, Co ordinates, Angle in Degrees, Text Size and Text Color for Overlay//\",\n                \"OverlayOptions\": {\n                  \"OverlayEnable\": true,\n                  \"OverlayText\": \"Collar Width\",\n                  \"OverlayCoords\": [\n                    5,\n                    8\n                  ],\n                  \"OverlayAngle\": 56,\n                  \"OverlayTextSize\": 6,\n                  \"OverlayTextColor\": \"Red\"\n                },\n                \"ResultVariable\": \"M1\"\n              },\n              {\n                \"AlgoName\": \"MoveXYTable\",\n                \"XYDelta\": [\n                  56,\n                  -33.8\n                ]\n              },\n              {\n                \"AlgoName\": \"MaxClamp\",\n                \"ThreadId\": 1,\n                \"ThreadImageId\": 2,\n                \"Option1\": \"\",\n                \"Option2\": \"\",\n                \"Option3\": \"\",\n                \"LocalRef\": {\n                  \"LocalCoordinateSystemEnable\": true,\n                  \"Method\": [\n                    \"A\",\n                    \"B\",\n                    \"C\",\n                    \"D\",\n                    \"R\",\n                    \"V\"\n                  ],\n                  \"ROIs\": [\n                    [\n                      23,\n                      78,\n                      99,\n                      25,\n                      0\n                    ],\n                    [\n                      67,\n                      97,\n                      43,\n                      9,\n                      0\n                    ],\n                    [\n                      45,\n                      88,\n                      723,\n                      85,\n                      0\n                    ]\n                  ],\n                  \"Name\": \"CollarWidthLocalReference\"\n                },\n                \"LocalROIs\": [\n                  [\n                    23,\n                    78,\n                    99,\n                    25,\n                    0\n                  ],\n                  [\n                    67,\n                    97,\n                    43,\n                    9,\n                    0\n                  ],\n                  [\n                    45,\n                    88,\n                    723,\n                    85,\n                    0\n                  ]\n                ],\n                \"comment_Overlay\": \"//OverlayOptions contain Text, Co ordinates, Angle in Degrees, Text Size and Text Color for Overlay//\",\n                \"OverlayOptions\": {\n                  \"OverlayEnable\": true,\n                  \"OverlayText\": \"Collar Width\",\n                  \"OverlayCoords\": [\n                    5,\n                    8\n                  ],\n                  \"OverlayAngle\": 56,\n                  \"OverlayTextSize\": 6,\n                  \"OverlayTextColor\": \"Red\"\n                },\n                \"ResultVariable\": \"M2\"\n              },\n              {\n                \"Algorithm\": \"Math\",\n                \"MathExpression\": \"M2-M1\",\n                \"ResultVariable\": \"M3\"\n              }\n            ],\n            \"CalibrationCoefficients\": [\n              13,\n              8.7,\n              67.9\n            ],\n            \"UserCorrectionLinearityCoeff\": 45,\n            \"UserCorrectionBiasCoeff\": 56,\n            \"comment_LSL\": \"//Lower Specification Limit//\",\n            \"LSL\": 13.5,\n            \"comment_USL\": \"//Upper Specification Limit//\",\n            \"USL\": 15,\n            \"comment_LCL\": \"//Lower Control Limit//\",\n            \"LCL\": 13.5,\n            \"comment_UCL\": \"//Upper Control Limit//\",\n            \"UCL\": 15,\n            \"comment_ControlLimitsViolationThreshold\": \"//If 3 measurement results out of 1000, are crossing LCL and UCL then fail is detected//\",\n            \"ControlLimitsViolationThreshold\": [\n              3,\n              1000\n            ],\n            \"comment_SpecificationLimitsViolationThreshold\": \"//If 5 measurement results out of 5000, are crossing LSL and USL then fail is detected//\",\n            \"SpecificationLimitViolationThreshold\": [\n              5,\n              5000\n            ],\n            \"comment_Overlay\": \"//OverlayOptions contain Text, Co ordinates, Angle in Degrees, Text Size and Text Color for Overlay//\",\n            \"OverlayOptions\": {\n              \"OverlayEnable\": true,\n              \"OverlayText\": \"Collar Width\",\n              \"OverlayCoords\": [\n                5,\n                8\n              ],\n              \"OverlayAngle\": 56,\n              \"OverlayTextSize\": 6,\n              \"OverlayTextColor\": \"Red\"\n            },\n            \"DatalogEnable\": true,\n            \"DisplayIcon\": \"C:\\\\Desktop\\\\displayimage.png\"\n          },\n          {\n            \"Name\": \"Length\",\n            \"comment_Type\": \"//Type can be Linear or Angle//\",\n            \"Type\": \"Linear\",\n            \"Enable\": true,\n            \"comment_AlgorithmSequence\": \"//Particular Measurement may require sequence of Algorithms. ThreadId and ThreadImageId are mentioned in each Algorithm which corresponds to particular combination of Camera and Light Ids. Result of each Algorithm is stored in a variable and final result is calculated using Math Expression defined.//\",\n            \"AlgorithmSequence\": [\n              {\n                \"AlgoName\": \"MaxClamp\",\n                \"ThreadId\": 1,\n                \"ThreadImageId\": 2,\n                \"Option1\": \"\",\n                \"Option2\": \"\",\n                \"Option3\": \"\",\n                \"LocalRef\": {\n                  \"LocalCoordinateSystemEnable\": true,\n                  \"Method\": [\n                    \"A\",\n                    \"B\",\n                    \"C\",\n                    \"D\",\n                    \"R\",\n                    \"V\"\n                  ],\n                  \"comment_LocalRefROI\": \"//Local Reference ROI is cluster of Left, Top, Right, Bottom and Rotation values//\",\n                  \"ROIs\": [\n                    [\n                      23,\n                      78,\n                      99,\n                      25,\n                      0\n                    ],\n                    [\n                      67,\n                      97,\n                      43,\n                      9,\n                      0\n                    ],\n                    [\n                      45,\n                      88,\n                      723,\n                      85,\n                      0\n                    ]\n                  ],\n                  \"Name\": \"CollarWidthLocalReference\"\n                },\n                \"LocalROIs\": [\n                  [\n                    23,\n                    78,\n                    99,\n                    25,\n                    0\n                  ],\n                  [\n                    67,\n                    97,\n                    43,\n                    9,\n                    0\n                  ],\n                  [\n                    45,\n                    88,\n                    723,\n                    85,\n                    0\n                  ]\n                ],\n                \"comment_Overlay\": \"//OverlayOptions contain Text, Co ordinates, Angle in Degrees, Text Size and Text Color for Overlay//\",\n                \"OverlayOptions\": {\n                  \"OverlayEnable\": true,\n                  \"OverlayText\": \"Collar Width\",\n                  \"OverlayCoords\": [\n                    5,\n                    8\n                  ],\n                  \"OverlayAngle\": 56,\n                  \"OverlayTextSize\": 6,\n                  \"OverlayTextColor\": \"Red\"\n                },\n                \"ResultVariable\": \"M1\"\n              },\n              {\n                \"AlgoName\": \"MoveXYTable\",\n                \"XYDelta\": [\n                  56,\n                  -33.8\n                ]\n              },\n              {\n                \"AlgoName\": \"MaxClamp\",\n                \"ThreadId\": 1,\n                \"ThreadImageId\": 2,\n                \"Option1\": \"\",\n                \"Option2\": \"\",\n                \"Option3\": \"\",\n                \"LocalRef\": {\n                  \"LocalCoordinateSystemEnable\": true,\n                  \"Method\": [\n                    \"A\",\n                    \"B\",\n                    \"C\",\n                    \"D\",\n                    \"R\",\n                    \"V\"\n                  ],\n                  \"ROIs\": [\n                    [\n                      23,\n                      78,\n                      99,\n                      25,\n                      0\n                    ],\n                    [\n                      67,\n                      97,\n                      43,\n                      9,\n                      0\n                    ],\n                    [\n                      45,\n                      88,\n                      723,\n                      85,\n                      0\n                    ]\n                  ],\n                  \"Name\": \"CollarWidthLocalReference\"\n                },\n                \"LocalROIs\": [\n                  [\n                    23,\n                    78,\n                    99,\n                    25,\n                    0\n                  ],\n                  [\n                    67,\n                    97,\n                    43,\n                    9,\n                    0\n                  ],\n                  [\n                    45,\n                    88,\n                    723,\n                    85,\n                    0\n                  ]\n                ],\n                \"comment_Overlay\": \"//OverlayOptions contain Text, Co ordinates, Angle in Degrees, Text Size and Text Color for Overlay//\",\n                \"OverlayOptions\": {\n                  \"OverlayEnable\": true,\n                  \"OverlayText\": \"Collar Width\",\n                  \"OverlayCoords\": [\n                    5,\n                    8\n                  ],\n                  \"OverlayAngle\": 56,\n                  \"OverlayTextSize\": 6,\n                  \"OverlayTextColor\": \"Red\"\n                },\n                \"ResultVariable\": \"M2\"\n              },\n              {\n                \"Algorithm\": \"Math\",\n                \"MathExpression\": \"M2-M1\",\n                \"ResultVariable\": \"M3\"\n              }\n            ],\n            \"CalibrationCoefficients\": [\n              13,\n              8.7,\n              67.9\n            ],\n            \"UserCorrectionLinearityCoeff\": 45,\n            \"UserCorrectionBiasCoeff\": 56,\n            \"comment_LSL\": \"//Lower Specification Limit//\",\n            \"LSL\": 13.5,\n            \"comment_USL\": \"//Upper Specification Limit//\",\n            \"USL\": 15,\n            \"comment_LCL\": \"//Lower Control Limit//\",\n            \"LCL\": 13.5,\n            \"comment_UCL\": \"//Upper Control Limit//\",\n            \"UCL\": 15,\n            \"comment_ControlLimitsViolationThreshold\": \"//If 3 measurement results out of 1000, are crossing LCL and UCL then fail is detected//\",\n            \"ControlLimitsViolationThreshold\": [\n              3,\n              1000\n            ],\n            \"comment_SpecificationLimitsViolationThreshold\": \"//If 5 measurement results out of 5000, are crossing LSL and USL then fail is detected//\",\n            \"SpecificationLimitViolationThreshold\": [\n              5,\n              5000\n            ],\n            \"comment_Overlay\": \"//OverlayOptions contain Text, Co ordinates, Angle in Degrees, Text Size and Text Color for Overlay//\",\n            \"OverlayOptions\": {\n              \"OverlayEnable\": true,\n              \"OverlayText\": \"Collar Width\",\n              \"OverlayCoords\": [\n                5,\n                8\n              ],\n              \"OverlayAngle\": 56,\n              \"OverlayTextSize\": 6,\n              \"OverlayTextColor\": \"Red\"\n            },\n            \"DatalogEnable\": true,\n            \"DisplayIcon\": \"C:\\\\Desktop\\\\displayimage.png\"\n          },\n          {\n            \"Name\": \"Length2\",\n            \"comment_Type\": \"//Type can be Linear or Angle//\",\n            \"Type\": \"Linear\",\n            \"Enable\": true,\n            \"comment_AlgorithmSequence\": \"//Particular Measurement may require sequence of Algorithms. ThreadId and ThreadImageId are mentioned in each Algorithm which corresponds to particular combination of Camera and Light Ids. Result of each Algorithm is stored in a variable and final result is calculated using Math Expression defined.//\",\n            \"AlgorithmSequence\": [\n              {\n                \"AlgoName\": \"MaxClamp\",\n                \"ThreadId\": 1,\n                \"ThreadImageId\": 2,\n                \"Option1\": \"\",\n                \"Option2\": \"\",\n                \"Option3\": \"\",\n                \"LocalRef\": {\n                  \"LocalCoordinateSystemEnable\": true,\n                  \"Method\": [\n                    \"A\",\n                    \"B\",\n                    \"C\",\n                    \"D\",\n                    \"R\",\n                    \"V\"\n                  ],\n                  \"comment_LocalRefROI\": \"//Local Reference ROI is cluster of Left, Top, Right, Bottom and Rotation values//\",\n                  \"ROIs\": [\n                    [\n                      23,\n                      78,\n                      99,\n                      25,\n                      0\n                    ],\n                    [\n                      67,\n                      97,\n                      43,\n                      9,\n                      0\n                    ],\n                    [\n                      45,\n                      88,\n                      723,\n                      85,\n                      0\n                    ]\n                  ],\n                  \"Name\": \"CollarWidthLocalReference\"\n                },\n                \"LocalROIs\": [\n                  [\n                    23,\n                    78,\n                    99,\n                    25,\n                    0\n                  ],\n                  [\n                    67,\n                    97,\n                    43,\n                    9,\n                    0\n                  ],\n                  [\n                    45,\n                    88,\n                    723,\n                    85,\n                    0\n                  ]\n                ],\n                \"comment_Overlay\": \"//OverlayOptions contain Text, Co ordinates, Angle in Degrees, Text Size and Text Color for Overlay//\",\n                \"OverlayOptions\": {\n                  \"OverlayEnable\": true,\n                  \"OverlayText\": \"Collar Width\",\n                  \"OverlayCoords\": [\n                    5,\n                    8\n                  ],\n                  \"OverlayAngle\": 56,\n                  \"OverlayTextSize\": 6,\n                  \"OverlayTextColor\": \"Red\"\n                },\n                \"ResultVariable\": \"M1\"\n              },\n              {\n                \"AlgoName\": \"MoveXYTable\",\n                \"XYDelta\": [\n                  56,\n                  -33.8\n                ]\n              },\n              {\n                \"AlgoName\": \"MaxClamp\",\n                \"ThreadId\": 1,\n                \"ThreadImageId\": 2,\n                \"Option1\": \"\",\n                \"Option2\": \"\",\n                \"Option3\": \"\",\n                \"LocalRef\": {\n                  \"LocalCoordinateSystemEnable\": true,\n                  \"Method\": [\n                    \"A\",\n                    \"B\",\n                    \"C\",\n                    \"D\",\n                    \"R\",\n                    \"V\"\n                  ],\n                  \"ROIs\": [\n                    [\n                      23,\n                      78,\n                      99,\n                      25,\n                      0\n                    ],\n                    [\n                      67,\n                      97,\n                      43,\n                      9,\n                      0\n                    ],\n                    [\n                      45,\n                      88,\n                      723,\n                      85,\n                      0\n                    ]\n                  ],\n                  \"Name\": \"CollarWidthLocalReference\"\n                },\n                \"LocalROIs\": [\n                  [\n                    23,\n                    78,\n                    99,\n                    25,\n                    0\n                  ],\n                  [\n                    67,\n                    97,\n                    43,\n                    9,\n                    0\n                  ],\n                  [\n                    45,\n                    88,\n                    723,\n                    85,\n                    0\n                  ]\n                ],\n                \"comment_Overlay\": \"//OverlayOptions contain Text, Co ordinates, Angle in Degrees, Text Size and Text Color for Overlay//\",\n                \"OverlayOptions\": {\n                  \"OverlayEnable\": true,\n                  \"OverlayText\": \"Collar Width\",\n                  \"OverlayCoords\": [\n                    5,\n                    8\n                  ],\n                  \"OverlayAngle\": 56,\n                  \"OverlayTextSize\": 6,\n                  \"OverlayTextColor\": \"Red\"\n                },\n                \"ResultVariable\": \"M2\"\n              },\n              {\n                \"Algorithm\": \"Math\",\n                \"MathExpression\": \"M2-M1\",\n                \"ResultVariable\": \"M3\"\n              }\n            ],\n            \"CalibrationCoefficients\": [\n              13,\n              8.7,\n              67.9\n            ],\n            \"UserCorrectionLinearityCoeff\": 45,\n            \"UserCorrectionBiasCoeff\": 56,\n            \"comment_LSL\": \"//Lower Specification Limit//\",\n            \"LSL\": 13.5,\n            \"comment_USL\": \"//Upper Specification Limit//\",\n            \"USL\": 15,\n            \"comment_LCL\": \"//Lower Control Limit//\",\n            \"LCL\": 13.5,\n            \"comment_UCL\": \"//Upper Control Limit//\",\n            \"UCL\": 15,\n            \"comment_ControlLimitsViolationThreshold\": \"//If 3 measurement results out of 1000, are crossing LCL and UCL then fail is detected//\",\n            \"ControlLimitsViolationThreshold\": [\n              3,\n              1000\n            ],\n            \"comment_SpecificationLimitsViolationThreshold\": \"//If 5 measurement results out of 5000, are crossing LSL and USL then fail is detected//\",\n            \"SpecificationLimitViolationThreshold\": [\n              5,\n              5000\n            ],\n            \"comment_Overlay\": \"//OverlayOptions contain Text, Co ordinates, Angle in Degrees, Text Size and Text Color for Overlay//\",\n            \"OverlayOptions\": {\n              \"OverlayEnable\": true,\n              \"OverlayText\": \"Collar Width\",\n              \"OverlayCoords\": [\n                5,\n                8\n              ],\n              \"OverlayAngle\": 56,\n              \"OverlayTextSize\": 6,\n              \"OverlayTextColor\": \"Red\"\n            },\n            \"DatalogEnable\": true,\n            \"DisplayIcon\": \"C:\\\\Desktop\\\\displayimage.png\"\n          }\n        ]\n      },\n      {\n        \"Name\": \"ECU1513\",\n        \"comment_ParallelTriggerThreads\": \"//ParallelTriggerThreads contain Thread Name, Thread Id and Imaging Views. Combination of Camera and Light(s) is defined in Imaging View along with Sensor to Light Delay (in micro seconds), Light to Camera Trigger Delay, Light Pulse Width and Reference Co-ordinate system. Each Imaging View is given a Name and unique ImageId. Camera and Light(s) are accessed by their unique Ids.//\",\n        \"ParallelTriggerThreads\": [\n          {\n            \"ThreadName\": \"TopRack\",\n            \"ThreadId\": 1,\n            \"ImagingViews\": [\n              {\n                \"ImageId\": 1,\n                \"ViewName\": \"TopProfileView\",\n                \"CameraId\": 3,\n                \"LightIds\": [\n                  1,\n                  4,\n                  5\n                ],\n                \"SensorToLightDelayinUSec\": 12,\n                \"LightToCameraTriggerDelay\": 24,\n                \"LightPulseWidth\": 123,\n                \"ReferenceCoordSystem\": {\n                  \"Method\": [\n                    \"A\",\n                    \"B\",\n                    \"C\",\n                    \"D\",\n                    \"R\",\n                    \"V\"\n                  ],\n                  \"comment_RefROI\": \"//Reference ROI is cluster of Left, Top, Right, Bottom and Rotation values//\",\n                  \"ROI1\": [\n                    1014,\n                    95,\n                    1290,\n                    520,\n                    0\n                  ],\n                  \"ROI2\": [\n                    740,\n                    70,\n                    1040,\n                    340,\n                    0\n                  ],\n                  \"ROI3\": [\n                    1060,\n                    88,\n                    723,\n                    85,\n                    0\n                  ],\n                  \"Name\": \"FirstReference\"\n                }\n              },\n              {\n                \"ImageId\": 2,\n                \"ViewName\": \"TopLightView\",\n                \"CameraId\": 2,\n                \"LightIds\": [\n                  2,\n                  3,\n                  5\n                ],\n                \"SensorToLightDelayinUSec\": 12,\n                \"LightToCameraTriggerDelay\": 24,\n                \"LightPulseWidth\": 123,\n                \"ReferenceCoordSystem\": {\n                  \"Method\": [\n                    \"A\",\n                    \"B\",\n                    \"C\",\n                    \"D\",\n                    \"R\",\n                    \"V\"\n                  ],\n                  \"comment_RefROI\": \"//Reference ROI is cluster of Left, Top, Right, Bottom and Rotation values//\",\n                  \"ROI1\": [\n                    1014,\n                    95,\n                    1290,\n                    520,\n                    0\n                  ],\n                  \"ROI2\": [\n                    740,\n                    70,\n                    1040,\n                    340,\n                    0\n                  ],\n                  \"ROI3\": [\n                    1060,\n                    88,\n                    723,\n                    85,\n                    0\n                  ],\n                  \"Name\": \"FirstReference\"\n                }\n              }\n            ]\n          },\n          {\n            \"ThreadName\": \"BottomRack\",\n            \"ThreadId\": 2,\n            \"ImagingViews\": [\n              {\n                \"ImageId\": 1,\n                \"ViewName\": \"TopProfileView\",\n                \"CameraId\": 3,\n                \"LightIds\": [\n                  1,\n                  4,\n                  5\n                ],\n                \"SensorToLightDelayinUSec\": 12,\n                \"LightToCameraTriggerDelay\": 24,\n                \"LightPulseWidth\": 123,\n                \"ReferenceCoordSystem\": {\n                  \"Method\": [\n                    \"A\",\n                    \"B\",\n                    \"C\",\n                    \"D\",\n                    \"R\",\n                    \"V\"\n                  ],\n                  \"comment_RefROI\": \"//Reference ROI is cluster of Left, Top, Right, Bottom and Rotation values//\",\n                  \"ROI1\": [\n                    1014,\n                    95,\n                    1290,\n                    520,\n                    0\n                  ],\n                  \"ROI2\": [\n                    740,\n                    70,\n                    1040,\n                    340,\n                    0\n                  ],\n                  \"ROI3\": [\n                    1060,\n                    88,\n                    723,\n                    85,\n                    0\n                  ],\n                  \"Name\": \"FirstReference\"\n                }\n              },\n              {\n                \"ImageId\": 2,\n                \"ViewName\": \"TopLightView\",\n                \"CameraId\": 2,\n                \"LightIds\": [\n                  2,\n                  3,\n                  5\n                ],\n                \"SensorToLightDelayinUSec\": 12,\n                \"LightToCameraTriggerDelay\": 24,\n                \"LightPulseWidth\": 123,\n                \"ReferenceCoordSystem\": {\n                  \"Method\": [\n                    \"A\",\n                    \"B\",\n                    \"C\",\n                    \"D\",\n                    \"R\",\n                    \"V\"\n                  ],\n                  \"comment_RefROI\": \"//Reference ROI is cluster of Left, Top, Right, Bottom and Rotation values//\",\n                  \"ROI1\": [\n                    1014,\n                    95,\n                    1290,\n                    520,\n                    0\n                  ],\n                  \"ROI2\": [\n                    740,\n                    70,\n                    1040,\n                    340,\n                    0\n                  ],\n                  \"ROI3\": [\n                    1060,\n                    88,\n                    723,\n                    85,\n                    0\n                  ],\n                  \"Name\": \"FirstReference\"\n                }\n              }\n            ]\n          },\n          {\n            \"ThreadName\": \"DentIdentification\",\n            \"ThreadId\": 3,\n            \"ImagingViews\": [\n              {\n                \"ImageId\": 1,\n                \"ViewName\": \"TopProfileView\",\n                \"CameraId\": 3,\n                \"LightIds\": [\n                  1,\n                  4,\n                  5\n                ],\n                \"SensorToLightDelayinUSec\": 12,\n                \"LightToCameraTriggerDelay\": 24,\n                \"LightPulseWidth\": 123,\n                \"ReferenceCoordSystem\": {\n                  \"Method\": [\n                    \"A\",\n                    \"B\",\n                    \"C\",\n                    \"D\",\n                    \"R\",\n                    \"V\"\n                  ],\n                  \"comment_RefROI\": \"//Reference ROI is cluster of Left, Top, Right, Bottom and Rotation values//\",\n                  \"ROI1\": [\n                    23,\n                    78,\n                    99,\n                    25,\n                    0\n                  ],\n                  \"ROI2\": [\n                    67,\n                    97,\n                    43,\n                    9,\n                    0\n                  ],\n                  \"ROI3\": [\n                    45,\n                    88,\n                    723,\n                    85,\n                    0\n                  ],\n                  \"Name\": \"FirstReference\"\n                }\n              }\n            ]\n          }\n        ],\n        \"Number of Measurements\": 3,\n        \"comment_Measurements\": \"//Measurements section contains Name, Type, Enable, Algorithm Sequence, Calibration Co-efficients, User Correction Linearity Coefficients, User Correction Bias Coefficients, LSL, USL, LCL, UCL, Control Limits Violation Threshold, Specification Limits Violation Threshold, Overlay Options, Datalog Enable, Display Icon path for each Measurement//\",\n        \"Measurements\": [\n          {\n            \"Name\": \"CollarWidth\",\n            \"comment_Type\": \"//Type can be Linear or Angle//\",\n            \"Type\": \"Linear\",\n            \"Enable\": true,\n            \"comment_AlgorithmSequence\": \"//Particular Measurement may require sequence of Algorithms. ThreadId and ThreadImageId are mentioned in each Algorithm which corresponds to particular combination of Camera and Light Ids. Result of each Algorithm is stored in a variable and final result is calculated using Math Expression defined.//\",\n            \"AlgorithmSequence\": [\n              {\n                \"AlgoName\": \"MaxClamp\",\n                \"ThreadId\": 1,\n                \"ThreadImageId\": 2,\n                \"Option1\": \"\",\n                \"Option2\": \"\",\n                \"Option3\": \"\",\n                \"LocalRef\": {\n                  \"LocalCoordinateSystemEnable\": true,\n                  \"Method\": [\n                    \"A\",\n                    \"B\",\n                    \"C\",\n                    \"D\",\n                    \"R\",\n                    \"V\"\n                  ],\n                  \"comment_LocalRefROI\": \"//Local Reference ROI is cluster of Left, Top, Right, Bottom and Rotation values//\",\n                  \"ROIs\": [\n                    [\n                      23,\n                      78,\n                      99,\n                      25,\n                      0\n                    ],\n                    [\n                      67,\n                      97,\n                      43,\n                      9,\n                      0\n                    ],\n                    [\n                      45,\n                      88,\n                      723,\n                      85,\n                      0\n                    ]\n                  ],\n                  \"Name\": \"CollarWidthLocalReference\"\n                },\n                \"LocalROIs\": [\n                  [\n                    23,\n                    78,\n                    99,\n                    25,\n                    0\n                  ],\n                  [\n                    67,\n                    97,\n                    43,\n                    9,\n                    0\n                  ],\n                  [\n                    45,\n                    88,\n                    723,\n                    85,\n                    0\n                  ]\n                ],\n                \"comment_Overlay\": \"//OverlayOptions contain Text, Co ordinates, Angle in Degrees, Text Size and Text Color for Overlay//\",\n                \"OverlayOptions\": {\n                  \"OverlayEnable\": true,\n                  \"OverlayText\": \"Collar Width\",\n                  \"OverlayCoords\": [\n                    5,\n                    8\n                  ],\n                  \"OverlayAngle\": 56,\n                  \"OverlayTextSize\": 6,\n                  \"OverlayTextColor\": \"Red\"\n                },\n                \"ResultVariable\": \"M1\"\n              },\n              {\n                \"AlgoName\": \"MoveXYTable\",\n                \"XYDelta\": [\n                  56,\n                  -33.8\n                ]\n              },\n              {\n                \"AlgoName\": \"MaxClamp\",\n                \"ThreadId\": 1,\n                \"ThreadImageId\": 2,\n                \"Option1\": \"\",\n                \"Option2\": \"\",\n                \"Option3\": \"\",\n                \"LocalRef\": {\n                  \"LocalCoordinateSystemEnable\": true,\n                  \"Method\": [\n                    \"A\",\n                    \"B\",\n                    \"C\",\n                    \"D\",\n                    \"R\",\n                    \"V\"\n                  ],\n                  \"ROIs\": [\n                    [\n                      23,\n                      78,\n                      99,\n                      25,\n                      0\n                    ],\n                    [\n                      67,\n                      97,\n                      43,\n                      9,\n                      0\n                    ],\n                    [\n                      45,\n                      88,\n                      723,\n                      85,\n                      0\n                    ]\n                  ],\n                  \"Name\": \"CollarWidthLocalReference\"\n                },\n                \"LocalROIs\": [\n                  [\n                    23,\n                    78,\n                    99,\n                    25,\n                    0\n                  ],\n                  [\n                    67,\n                    97,\n                    43,\n                    9,\n                    0\n                  ],\n                  [\n                    45,\n                    88,\n                    723,\n                    85,\n                    0\n                  ]\n                ],\n                \"comment_Overlay\": \"//OverlayOptions contain Text, Co ordinates, Angle in Degrees, Text Size and Text Color for Overlay//\",\n                \"OverlayOptions\": {\n                  \"OverlayEnable\": true,\n                  \"OverlayText\": \"Collar Width\",\n                  \"OverlayCoords\": [\n                    5,\n                    8\n                  ],\n                  \"OverlayAngle\": 56,\n                  \"OverlayTextSize\": 6,\n                  \"OverlayTextColor\": \"Red\"\n                },\n                \"ResultVariable\": \"M2\"\n              },\n              {\n                \"Algorithm\": \"Math\",\n                \"MathExpression\": \"M2-M1\",\n                \"ResultVariable\": \"M3\"\n              }\n            ],\n            \"CalibrationCoefficients\": [\n              13,\n              8.7,\n              67.9\n            ],\n            \"UserCorrectionLinearityCoeff\": 45,\n            \"UserCorrectionBiasCoeff\": 56,\n            \"comment_LSL\": \"//Lower Specification Limit//\",\n            \"LSL\": 13.5,\n            \"comment_USL\": \"//Upper Specification Limit//\",\n            \"USL\": 15,\n            \"comment_LCL\": \"//Lower Control Limit//\",\n            \"LCL\": 13.5,\n            \"comment_UCL\": \"//Upper Control Limit//\",\n            \"UCL\": 15,\n            \"comment_ControlLimitsViolationThreshold\": \"//If 3 measurement results out of 1000, are crossing LCL and UCL then fail is detected//\",\n            \"ControlLimitsViolationThreshold\": [\n              3,\n              1000\n            ],\n            \"comment_SpecificationLimitsViolationThreshold\": \"//If 5 measurement results out of 5000, are crossing LSL and USL then fail is detected//\",\n            \"SpecificationLimitViolationThreshold\": [\n              5,\n              5000\n            ],\n            \"comment_Overlay\": \"//OverlayOptions contain Text, Co ordinates, Angle in Degrees, Text Size and Text Color for Overlay//\",\n            \"OverlayOptions\": {\n              \"OverlayEnable\": true,\n              \"OverlayText\": \"Collar Width\",\n              \"OverlayCoords\": [\n                5,\n                8\n              ],\n              \"OverlayAngle\": 56,\n              \"OverlayTextSize\": 6,\n              \"OverlayTextColor\": \"Red\"\n            },\n            \"DatalogEnable\": true,\n            \"DisplayIcon\": \"C:\\\\Desktop\\\\displayimage.png\"\n          },\n          {\n            \"Name\": \"Length\",\n            \"comment_Type\": \"//Type can be Linear or Angle//\",\n            \"Type\": \"Linear\",\n            \"Enable\": true,\n            \"comment_AlgorithmSequence\": \"//Particular Measurement may require sequence of Algorithms. ThreadId and ThreadImageId are mentioned in each Algorithm which corresponds to particular combination of Camera and Light Ids. Result of each Algorithm is stored in a variable and final result is calculated using Math Expression defined.//\",\n            \"AlgorithmSequence\": [\n              {\n                \"AlgoName\": \"MaxClamp\",\n                \"ThreadId\": 1,\n                \"ThreadImageId\": 2,\n                \"Option1\": \"\",\n                \"Option2\": \"\",\n                \"Option3\": \"\",\n                \"LocalRef\": {\n                  \"LocalCoordinateSystemEnable\": true,\n                  \"Method\": [\n                    \"A\",\n                    \"B\",\n                    \"C\",\n                    \"D\",\n                    \"R\",\n                    \"V\"\n                  ],\n                  \"comment_LocalRefROI\": \"//Local Reference ROI is cluster of Left, Top, Right, Bottom and Rotation values//\",\n                  \"ROIs\": [\n                    [\n                      23,\n                      78,\n                      99,\n                      25,\n                      0\n                    ],\n                    [\n                      67,\n                      97,\n                      43,\n                      9,\n                      0\n                    ],\n                    [\n                      45,\n                      88,\n                      723,\n                      85,\n                      0\n                    ]\n                  ],\n                  \"Name\": \"CollarWidthLocalReference\"\n                },\n                \"LocalROIs\": [\n                  [\n                    23,\n                    78,\n                    99,\n                    25,\n                    0\n                  ],\n                  [\n                    67,\n                    97,\n                    43,\n                    9,\n                    0\n                  ],\n                  [\n                    45,\n                    88,\n                    723,\n                    85,\n                    0\n                  ]\n                ],\n                \"comment_Overlay\": \"//OverlayOptions contain Text, Co ordinates, Angle in Degrees, Text Size and Text Color for Overlay//\",\n                \"OverlayOptions\": {\n                  \"OverlayEnable\": true,\n                  \"OverlayText\": \"Collar Width\",\n                  \"OverlayCoords\": [\n                    5,\n                    8\n                  ],\n                  \"OverlayAngle\": 56,\n                  \"OverlayTextSize\": 6,\n                  \"OverlayTextColor\": \"Red\"\n                },\n                \"ResultVariable\": \"M1\"\n              },\n              {\n                \"AlgoName\": \"MoveXYTable\",\n                \"XYDelta\": [\n                  56,\n                  -33.8\n                ]\n              },\n              {\n                \"AlgoName\": \"MaxClamp\",\n                \"ThreadId\": 1,\n                \"ThreadImageId\": 2,\n                \"Option1\": \"\",\n                \"Option2\": \"\",\n                \"Option3\": \"\",\n                \"LocalRef\": {\n                  \"LocalCoordinateSystemEnable\": true,\n                  \"Method\": [\n                    \"A\",\n                    \"B\",\n                    \"C\",\n                    \"D\",\n                    \"R\",\n                    \"V\"\n                  ],\n                  \"ROIs\": [\n                    [\n                      23,\n                      78,\n                      99,\n                      25,\n                      0\n                    ],\n                    [\n                      67,\n                      97,\n                      43,\n                      9,\n                      0\n                    ],\n                    [\n                      45,\n                      88,\n                      723,\n                      85,\n                      0\n                    ]\n                  ],\n                  \"Name\": \"CollarWidthLocalReference\"\n                },\n                \"LocalROIs\": [\n                  [\n                    23,\n                    78,\n                    99,\n                    25,\n                    0\n                  ],\n                  [\n                    67,\n                    97,\n                    43,\n                    9,\n                    0\n                  ],\n                  [\n                    45,\n                    88,\n                    723,\n                    85,\n                    0\n                  ]\n                ],\n                \"comment_Overlay\": \"//OverlayOptions contain Text, Co ordinates, Angle in Degrees, Text Size and Text Color for Overlay//\",\n                \"OverlayOptions\": {\n                  \"OverlayEnable\": true,\n                  \"OverlayText\": \"Collar Width\",\n                  \"OverlayCoords\": [\n                    5,\n                    8\n                  ],\n                  \"OverlayAngle\": 56,\n                  \"OverlayTextSize\": 6,\n                  \"OverlayTextColor\": \"Red\"\n                },\n                \"ResultVariable\": \"M2\"\n              },\n              {\n                \"Algorithm\": \"Math\",\n                \"MathExpression\": \"M2-M1\",\n                \"ResultVariable\": \"M3\"\n              }\n            ],\n            \"CalibrationCoefficients\": [\n              13,\n              8.7,\n              67.9\n            ],\n            \"UserCorrectionLinearityCoeff\": 45,\n            \"UserCorrectionBiasCoeff\": 56,\n            \"comment_LSL\": \"//Lower Specification Limit//\",\n            \"LSL\": 13.5,\n            \"comment_USL\": \"//Upper Specification Limit//\",\n            \"USL\": 15,\n            \"comment_LCL\": \"//Lower Control Limit//\",\n            \"LCL\": 13.5,\n            \"comment_UCL\": \"//Upper Control Limit//\",\n            \"UCL\": 15,\n            \"comment_ControlLimitsViolationThreshold\": \"//If 3 measurement results out of 1000, are crossing LCL and UCL then fail is detected//\",\n            \"ControlLimitsViolationThreshold\": [\n              3,\n              1000\n            ],\n            \"comment_SpecificationLimitsViolationThreshold\": \"//If 5 measurement results out of 5000, are crossing LSL and USL then fail is detected//\",\n            \"SpecificationLimitViolationThreshold\": [\n              5,\n              5000\n            ],\n            \"comment_Overlay\": \"//OverlayOptions contain Text, Co ordinates, Angle in Degrees, Text Size and Text Color for Overlay//\",\n            \"OverlayOptions\": {\n              \"OverlayEnable\": true,\n              \"OverlayText\": \"Collar Width\",\n              \"OverlayCoords\": [\n                5,\n                8\n              ],\n              \"OverlayAngle\": 56,\n              \"OverlayTextSize\": 6,\n              \"OverlayTextColor\": \"Red\"\n            },\n            \"DatalogEnable\": true,\n            \"DisplayIcon\": \"C:\\\\Desktop\\\\displayimage.png\"\n          },\n          {\n            \"Name\": \"Length2\",\n            \"comment_Type\": \"//Type can be Linear or Angle//\",\n            \"Type\": \"Linear\",\n            \"Enable\": true,\n            \"comment_AlgorithmSequence\": \"//Particular Measurement may require sequence of Algorithms. ThreadId and ThreadImageId are mentioned in each Algorithm which corresponds to particular combination of Camera and Light Ids. Result of each Algorithm is stored in a variable and final result is calculated using Math Expression defined.//\",\n            \"AlgorithmSequence\": [\n              {\n                \"AlgoName\": \"MaxClamp\",\n                \"ThreadId\": 1,\n                \"ThreadImageId\": 2,\n                \"Option1\": \"\",\n                \"Option2\": \"\",\n                \"Option3\": \"\",\n                \"LocalRef\": {\n                  \"LocalCoordinateSystemEnable\": true,\n                  \"Method\": [\n                    \"A\",\n                    \"B\",\n                    \"C\",\n                    \"D\",\n                    \"R\",\n                    \"V\"\n                  ],\n                  \"comment_LocalRefROI\": \"//Local Reference ROI is cluster of Left, Top, Right, Bottom and Rotation values//\",\n                  \"ROIs\": [\n                    [\n                      23,\n                      78,\n                      99,\n                      25,\n                      0\n                    ],\n                    [\n                      67,\n                      97,\n                      43,\n                      9,\n                      0\n                    ],\n                    [\n                      45,\n                      88,\n                      723,\n                      85,\n                      0\n                    ]\n                  ],\n                  \"Name\": \"CollarWidthLocalReference\"\n                },\n                \"LocalROIs\": [\n                  [\n                    23,\n                    78,\n                    99,\n                    25,\n                    0\n                  ],\n                  [\n                    67,\n                    97,\n                    43,\n                    9,\n                    0\n                  ],\n                  [\n                    45,\n                    88,\n                    723,\n                    85,\n                    0\n                  ]\n                ],\n                \"comment_Overlay\": \"//OverlayOptions contain Text, Co ordinates, Angle in Degrees, Text Size and Text Color for Overlay//\",\n                \"OverlayOptions\": {\n                  \"OverlayEnable\": true,\n                  \"OverlayText\": \"Collar Width\",\n                  \"OverlayCoords\": [\n                    5,\n                    8\n                  ],\n                  \"OverlayAngle\": 56,\n                  \"OverlayTextSize\": 6,\n                  \"OverlayTextColor\": \"Red\"\n                },\n                \"ResultVariable\": \"M1\"\n              },\n              {\n                \"AlgoName\": \"MoveXYTable\",\n                \"XYDelta\": [\n                  56,\n                  -33.8\n                ]\n              },\n              {\n                \"AlgoName\": \"MaxClamp\",\n                \"ThreadId\": 1,\n                \"ThreadImageId\": 2,\n                \"Option1\": \"\",\n                \"Option2\": \"\",\n                \"Option3\": \"\",\n                \"LocalRef\": {\n                  \"LocalCoordinateSystemEnable\": true,\n                  \"Method\": [\n                    \"A\",\n                    \"B\",\n                    \"C\",\n                    \"D\",\n                    \"R\",\n                    \"V\"\n                  ],\n                  \"ROIs\": [\n                    [\n                      23,\n                      78,\n                      99,\n                      25,\n                      0\n                    ],\n                    [\n                      67,\n                      97,\n                      43,\n                      9,\n                      0\n                    ],\n                    [\n                      45,\n                      88,\n                      723,\n                      85,\n                      0\n                    ]\n                  ],\n                  \"Name\": \"CollarWidthLocalReference\"\n                },\n                \"LocalROIs\": [\n                  [\n                    23,\n                    78,\n                    99,\n                    25,\n                    0\n                  ],\n                  [\n                    67,\n                    97,\n                    43,\n                    9,\n                    0\n                  ],\n                  [\n                    45,\n                    88,\n                    723,\n                    85,\n                    0\n                  ]\n                ],\n                \"comment_Overlay\": \"//OverlayOptions contain Text, Co ordinates, Angle in Degrees, Text Size and Text Color for Overlay//\",\n                \"OverlayOptions\": {\n                  \"OverlayEnable\": true,\n                  \"OverlayText\": \"Collar Width\",\n                  \"OverlayCoords\": [\n                    5,\n                    8\n                  ],\n                  \"OverlayAngle\": 56,\n                  \"OverlayTextSize\": 6,\n                  \"OverlayTextColor\": \"Red\"\n                },\n                \"ResultVariable\": \"M2\"\n              },\n              {\n                \"Algorithm\": \"Math\",\n                \"MathExpression\": \"M2-M1\",\n                \"ResultVariable\": \"M3\"\n              }\n            ],\n            \"CalibrationCoefficients\": [\n              13,\n              8.7,\n              67.9\n            ],\n            \"UserCorrectionLinearityCoeff\": 45,\n            \"UserCorrectionBiasCoeff\": 56,\n            \"comment_LSL\": \"//Lower Specification Limit//\",\n            \"LSL\": 13.5,\n            \"comment_USL\": \"//Upper Specification Limit//\",\n            \"USL\": 15,\n            \"comment_LCL\": \"//Lower Control Limit//\",\n            \"LCL\": 13.5,\n            \"comment_UCL\": \"//Upper Control Limit//\",\n            \"UCL\": 15,\n            \"comment_ControlLimitsViolationThreshold\": \"//If 3 measurement results out of 1000, are crossing LCL and UCL then fail is detected//\",\n            \"ControlLimitsViolationThreshold\": [\n              3,\n              1000\n            ],\n            \"comment_SpecificationLimitsViolationThreshold\": \"//If 5 measurement results out of 5000, are crossing LSL and USL then fail is detected//\",\n            \"SpecificationLimitViolationThreshold\": [\n              5,\n              5000\n            ],\n            \"comment_Overlay\": \"//OverlayOptions contain Text, Co ordinates, Angle in Degrees, Text Size and Text Color for Overlay//\",\n            \"OverlayOptions\": {\n              \"OverlayEnable\": true,\n              \"OverlayText\": \"Collar Width\",\n              \"OverlayCoords\": [\n                5,\n                8\n              ],\n              \"OverlayAngle\": 56,\n              \"OverlayTextSize\": 6,\n              \"OverlayTextColor\": \"Red\"\n            },\n            \"DatalogEnable\": true,\n            \"DisplayIcon\": \"C:\\\\Desktop\\\\displayimage.png\"\n          }\n        ]\n      }\n    ]\n  },\n  \"AlgoParameters\": {\n    \"comment_RefROIEdgeOptions\": \"Reference ROI Edge Options is cluster of Edge Polarity, Kernel Size, Width, Minimum Edge Strength, Interpolation Type and Data Processing Method\",\n    \"RefROIEdgeOptions\": [\n      0,\n      2,\n      3,\n      3,\n      50,\n      0\n    ],\n    \"comment_RefROILineOptions\": \"Reference ROI Line Options is cluster of Number of lines, Type, Min. score, Max Score Orientation, Angle Range, Angle Tolerance, Step size, Min. SNR(db), Min Points (%) and Hough Iterations\",\n    \"RefROILineOptions\": [\n      1,\n      1,\n      10,\n      1000,\n      0,\n      10,\n      1,\n      10,\n      0,\n      25\n    ],\n    \"StepSize\": 14\n  }\n}" ("JSON String")
  # "Can use this for testing"
  n1 = case shown="No Error" "error in" {
    selector: "error in" -> [w13 w235]
    tunnel: [w17 w235] -> w5
    tunnel: "Type and Defaults" -> [w10 _]
    tunnel: "basePath in" -> [w9 _]
    tunnel: "JSON String" -> [w8 _]
    tunnel: "pathList" -> [w7 _]
    frame No Error {
      n2 = call "basePath.vi"("error in (no error)"=w13, "pathList"=w7, "basePath in"=w9) -> ("error out"=w12:errorcluster, "pathArray out"=w11:string[])  [unwired: 7 in]
      n3 = for {
        tunnel: w11 -> [w19] mode=indexing
        tunnel: w8 -> [w26]
        shift-right: [w21] -> w16
        shift-left: w12 -> [w25]
        tunnel: [w20] -> w15 mode=indexing
        tunnel: w10 -> [w18]
        # "Get each and every JSONpath element one by one given in ArrayOfPaths"
        n4 = call <vilib>:"Unflatten From JSON String.vi"("Type and Defaults"=w18, "error in (no error)"=w25, "JSON String"=w26) -> ("error out"=w27:errorcluster, "Variant"=w24:variant)  [unwired: 7 in]
        n5 = call "jsonPath.vi"("error in (no error)"=w27, "json path in"=w19) -> ("error out"=w22:errorcluster, "output array of keys"=w23:string[])  [unwired: 8 in]
        n6 = for {
          tunnel: w23 -> [w40] mode=indexing
          shift-right: [w47] -> w20
          shift-left: w24 -> [w33]
          shift-right: [w45] -> w21
          shift-left: w22 -> [w46]
          tunnel: w19 -> [w29]
          stop <- w28 stop-if-true
          # "Get into respective Clusters/Arrays"
          n7 = call <vilib>:"Get Type Information.vi"("Variant"=w33) -> ("Type"=w32:T1)  [unwired: 6 in, 4 out]
          n8 = Search/Split String(string=w40, search string/char (-)="[") -> (offset of match=w41:i32)  [unwired: 1 in, 2 out]
          n9 = xnode "Match Regular Expression"("input string"=w40, "regular expression"="\\[") -> ("before match"=w43:string, "after match"=w38:string)  [unwired: 4 in, 3 out]
          n10 = Equal?(x=w32, y=Data_Type."Array") -> (x = y?=w30:bool)
          n11 = Equal?(x=w38, y="]") -> (x = y?=w37:bool)
          n12 = Not(x=w37) -> (.not. x?=w34:bool)
          n13 = Not Equal?(x=w41, y=-1) -> (x != y?=w36:bool)
          n14 = And(x=w34, y=w36) -> (x .and. y?=w35:bool)
          n15 = case shown="True" w30 {
            tunnel: [w57 w97] -> w47
            tunnel: w46 -> [w56 w95]
            tunnel: [w55 w94] -> w45
            tunnel: w43 -> [w54 _]
            tunnel: w40 -> [w53 w100]
            tunnel: w35 -> [w52 _]
            tunnel: w34 -> [w51 _]
            tunnel: w33 -> [w50 w102]
            tunnel: w29 -> [_ w101]
            tunnel: [FALSE w96] -> w28
            frame False {
              # "Gives particular elements pertaining to a cluster"
              n16 = case shown="False" w52 {
                tunnel: w50 -> [w65 w75]
                tunnel: [w64 w80] -> w57
                tunnel: w53 -> [w60 w68]
                tunnel: w56 -> [w63 w70]
                tunnel: [w62 w79] -> w55
                tunnel: w54 -> [w58 w73]
                tunnel: w51 -> [w61 _]
                frame False {
                  # "Retreive cluster element values using input string path"
                  n17 = case shown="False" w61 {
                    tunnel: w60 -> [_ w67]
                    tunnel: [w66 w67] -> w59
                    tunnel: w58 -> [w66 _]
                    frame False {
                      # "contains the \"[]\"\nso remove the square brackets"
                    }
                    frame True {
                      # "does not contain \"[]\"\nso pass the path as it is"
                    }
                  }
                  n18 = call <userlib>:"Get Cluster Element by Name__ogtk.vi"("error in (no error)"=w63, "Element Name"=w59, "Cluster"=w65) -> ("error out"=w62:errorcluster, "VElement"=w64:variant)  [unwired: 6 in, 1 out]
                }
                frame True {
                  # "Retreive array elements using input string path"
                  n19 = call "getKeyOrIndex.vi"("error in (no error)"=w70, "input string"=w68) -> ("error out"=w69:errorcluster, "value"=w76:string, "key"=w77:string, "index"=w78:i32, "keygiven?"=w71:bool)  [unwired: 5 in]
                  n20 = call <userlib>:"Get Cluster Element by Name__ogtk.vi"("error in (no error)"=w69, "Element Name"=w73, "Cluster"=w75) -> ("error out"=w72:errorcluster, "VElement"=w74:variant)  [unwired: 6 in, 1 out]
                  n21 = case shown="False" w71 {
                    tunnel: [w85 w86] -> w80
                    tunnel: [w84 w87] -> w79
                    tunnel: w74 -> [w83 w89]
                    tunnel: w72 -> [w82 w92]
                    tunnel: w78 -> [w81 _]
                    tunnel: w77 -> [_ w93]
                    tunnel: w76 -> [_ w91]
                    frame False {
                      # "key given"
                      n22 = call <userlib>:"Index Array__ogtk.vi"("error in (no error)"=w82, "Index (1D)"=w81, "MultiD Array"=w83) -> ("error out"=w84:errorcluster, "Array Element"=w85:variant)  [unwired: 7 in]
                    }
                    frame True {
                      # "Check for keys"
                      n23 = call "getIndex.vi"("error in (no error)"=w92, "value"=w91, "key"=w93, "VElement"=w89) -> ("error out"=w88:errorcluster, "indexOut"=w90:i32)  [unwired: 6 in]
                      n24 = call <userlib>:"Index Array__ogtk.vi"("error in (no error)"=w88, "Index (1D)"=w90, "MultiD Array"=w89) -> ("error out"=w87:errorcluster, "Array Element"=w86:variant)  [unwired: 7 in]
                    }
                  }
                }
              }
            }
            frame True {
              # "gives all the instances of an element in the same cluster but in different indices pertaining to an array."
              n25 = Search/Split String(string=w101, search string/char (-)=w100) -> (match + rest of string=w99:string)  [unwired: 1 in, 2 out]
              n26 = while {
                tunnel: w102 -> [w120]
                tunnel: w101 -> [_]
                tunnel: w99 -> [w115]
                tunnel: [w105] -> w98 mode=indexing
                tunnel: [w112] -> w96
                tunnel: w95 -> [w111]
                tunnel: [w103] -> w94
                i -> [w114]
                stop <- w112 stop-if-true
                n27 = call <userlib>:"Array Size(s)__ogtk.vi"("error in (no error)"=w111, "Array"=w120) -> ("error out"=w110:errorcluster, "Size(s)"=w119:u32[])  [unwired: 7 in, 1 out]
                n28 = Concatenate Strings("$." ("string"), w115) -> (w107:string)
                n29 = Increment(x=w114) -> (x+1=w113:i32)
                n30 = Index Array(array=w119) -> (element=w118:u32)  [unwired: 1 in]
                n31 = call <userlib>:"Index Array__ogtk.vi"("error in (no error)"=w110, "Index (1D)"=w114, "MultiD Array"=w120) -> ("error out"=w109:errorcluster, "Array Element"=w117:variant)  [unwired: 7 in]
                n32 = Equal?(x=w118, y=w113) -> (x = y?=w112:bool)
                n33 = call <vilib>:"Flatten To JSON String.vi"("error in (no error)"=w109, "Variant"=w117) -> ("error out"=w104:errorcluster, "JSON String"=w108:string)  [unwired: 8 in]
                n34 = Build Array(w107) -> (w106:string[])
                n35 = call "mainSingleCodeTestBench2.vi"("error in"=w104, "pathList"=w106, "JSON String"=w108) -> ("error out"=w103:errorcluster, "VClusterOut"=w105:variant)  [unwired: 7 in]
              }
              n36 = call <userlib>:"Array of VData to VArray__ogtk.vi"("1D Array of VData"=w98) -> ("VArray"=w97:variant)  [unwired: 9 in, 1 out]
            }
          }
        }
      }
      n37 = call <userlib>:"Array to VCluster__ogtk.vi"("error in (no error)"=w16, "Array"=w15) -> ("error out"=w17:errorcluster, "VCluster"=→"VClusterOut":variant)  [unwired: 8 in]
    }
    frame Error {
    }
  }
  "error out" <- w5
